vi "STED Control V11.vi"() -> ()   [LabVIEW 2014]
uses:
  Type Defs/Image Acquisition Parameters.ctl
  Laser Controls.ctl
  Detectors.ctl
  Type Defs/P541.ctl
  Type Defs/M227.ctl
  Type Defs/P612.ctl
  Type Defs/M686.ctl
  Type Defs/P841.ctl
  Type Defs/ASI.ctl
  Type Defs/N664_V2.ctl
  Type Defs/STED Graph Controls.ctl
  Type Defs/Display Controls.ctl
  FPGA-7842R-Reference.ctl
  Manual Controls V2.ctl
  Scan Parameters.ctl
  <vilib>/Utility/miscctls.llb/LVPositionTypeDef.ctl
  Focus Lock/Controls/Counter Action.ctl
  Controls/StageStates.ctl
  Focus Lock/Controls/Standard Action for Focus Lock.ctl
  <vilib>/Utility/miscctls.llb/LVRectTypeDef.ctl
  <vilib>/event_ctls.llb/lveventtype.ctl
  <vilib>/Utility/file.llb/Read From Spreadsheet File (DBL).vi
  <vilib>/Utility/file.llb/Write To Spreadsheet File (DBL).vi
panel:
  out "Graph Ref Out":refnum<vi>[](array[refnum])
  out "Frame Counter":i32
  in  "Follow Cursor":bool
  in  "Laser Controls 2":T1={"Laser On Time (Ticks)"=16, "Laser Delay (Ticks)"=3}
  out "Channel 6":sgl[][](graph)
  out "Channel 5":sgl[][](graph)
  out "Channel 4":sgl[][](graph)
  out "Channel 3":sgl[][](graph)
  out "Channel 2":sgl[][](graph)
  out "Channel 1":sgl[][](graph)
  in  "Display Controls":T2
  in  "Graph Tools":T3={"Zoom Out"=FALSE, "Zoom In"=FALSE, "Reset Zoom"=FALSE, "Pan Tool"=FALSE, "Show Cursor"=FALSE, "Load File"=FALSE, "Fit Tool"=FALSE, "Smooth Tool"=FALSE, "Merge Tool"=FALSE, "Auto Scale"=FALSE, "Apply Color"=FALSE, "Color Map"=enum."Fire"}
  in  "Shutters":T4
  in  "Upper Objective Z - N664":T5={"Up N664"=FALSE, "Down N664"=FALSE, "Step Size (um)"=0.001, "Position (mm)"=0.0, "Home"=FALSE, "Save"=FALSE} {"Step Size (um)" min=0.001}
  in  "Cavity Translation Z - ASI":T6={"Up ASI"=FALSE, "Down ASI"=FALSE, "Step Size (um)"=0.001, "Z (um)"=0.001, "F (um)"=0.001, "Velocity"=0.001} caption="ASI" {"Velocity" min=0.001; "F (um)" min=0.001; "Z (um)" min=-1500.0 max=1500.0; "Step Size (um)" min=0.001}
  in  "Phase Comp Mirror - P841":T7={"Position (µm)"=0.0, "Step Size (µm)"=0.05, "Up P841"=FALSE, "Down P841"=FALSE}
  in  "Sample Stage XY - M686":T8={"Home Button"=FALSE, "Up Button"=FALSE, "Left Button"=FALSE, "Down Button"=FALSE, "Right Button"=FALSE, "X"=0.0, "Y"=0.0, "Step Size (um)"=1.0} {"Y" format="%#_8g"; "X" format="%#_8g"}
  in  "Bottom Objective XY - P612":T9
  in  "Abort AllStage":bool
  in  "Stages":T10={"M227"=TRUE, "N664"=TRUE, "P612"=TRUE, "M686"=TRUE, "P841"=TRUE, "ASI"=FALSE}
  in  "Sample Z Coarse - M227":T11
  in  "Tab Control":T12(tab)
  in  "SLM":bool
  in  "DM":bool
  in  "Timing":bool
  in  "Focus Lock":bool
  in  "Stage Monitor":bool
  in  "Camera":bool
  in  "Sample Z - P541":T13={"Step Up"=FALSE, "Step Down"=FALSE, "Z Position"=0.0, "Step Size (um)"=1.0, "Home"=FALSE, "Save"=FALSE}
  in  "Detectors":T14={"PMT"=TRUE, "Far Red (685/40 nm)"=FALSE, "Orange (624/40 nm)"=FALSE, "Green (525/50 nm)"=FALSE, "Sum All"=FALSE}
  in  "Laser Controls":T15 {"STED Power (V)" scale=0.0..10.0}
  in  "Save File Path":path=path "C:/isoSTED_Data/Temp/Test_0000.dbl"
  in  "Capture":bool
  in  "Image Acquisition Parameters":T16={"Scan Type"=enum."Beam Scanning", "Scan Mode"=enum."XY", "Fast Axis Frequency (Hz)"=15780.0, "Image Format"=256, "Line Accumulations"=100, "Frames Per Capture"=1, "Frames Accumulations"=1, "Image Dimension (um)"=[15.0, 15.0], "Number of Z Steps"=1, "Z Steps Size (um)"=1.0, "Pixel Size (nm)"=[58.59375, 58.59375], "Customized Image Format"=[]} {"Z Steps Size (um)" min=0.0; "Number of Z Steps" min=1; "Frames Accumulations" min=1; "Frames Per Capture" min=1; "Line Accumulations" min=1; "Image Format" items=["64 x 64"=64, "128 x 128"=128, "256 x 256"=256, "512 x 512"=512, "1024 x 1024"=1024, "2048 x 2048"=2048, "Customized..."=0]}
  in  "Live":bool
  in  "Exit":bool
  # "Length"
  # "Height"
  # "XY"
  # "Z"
  # "Length"
  # "Height"
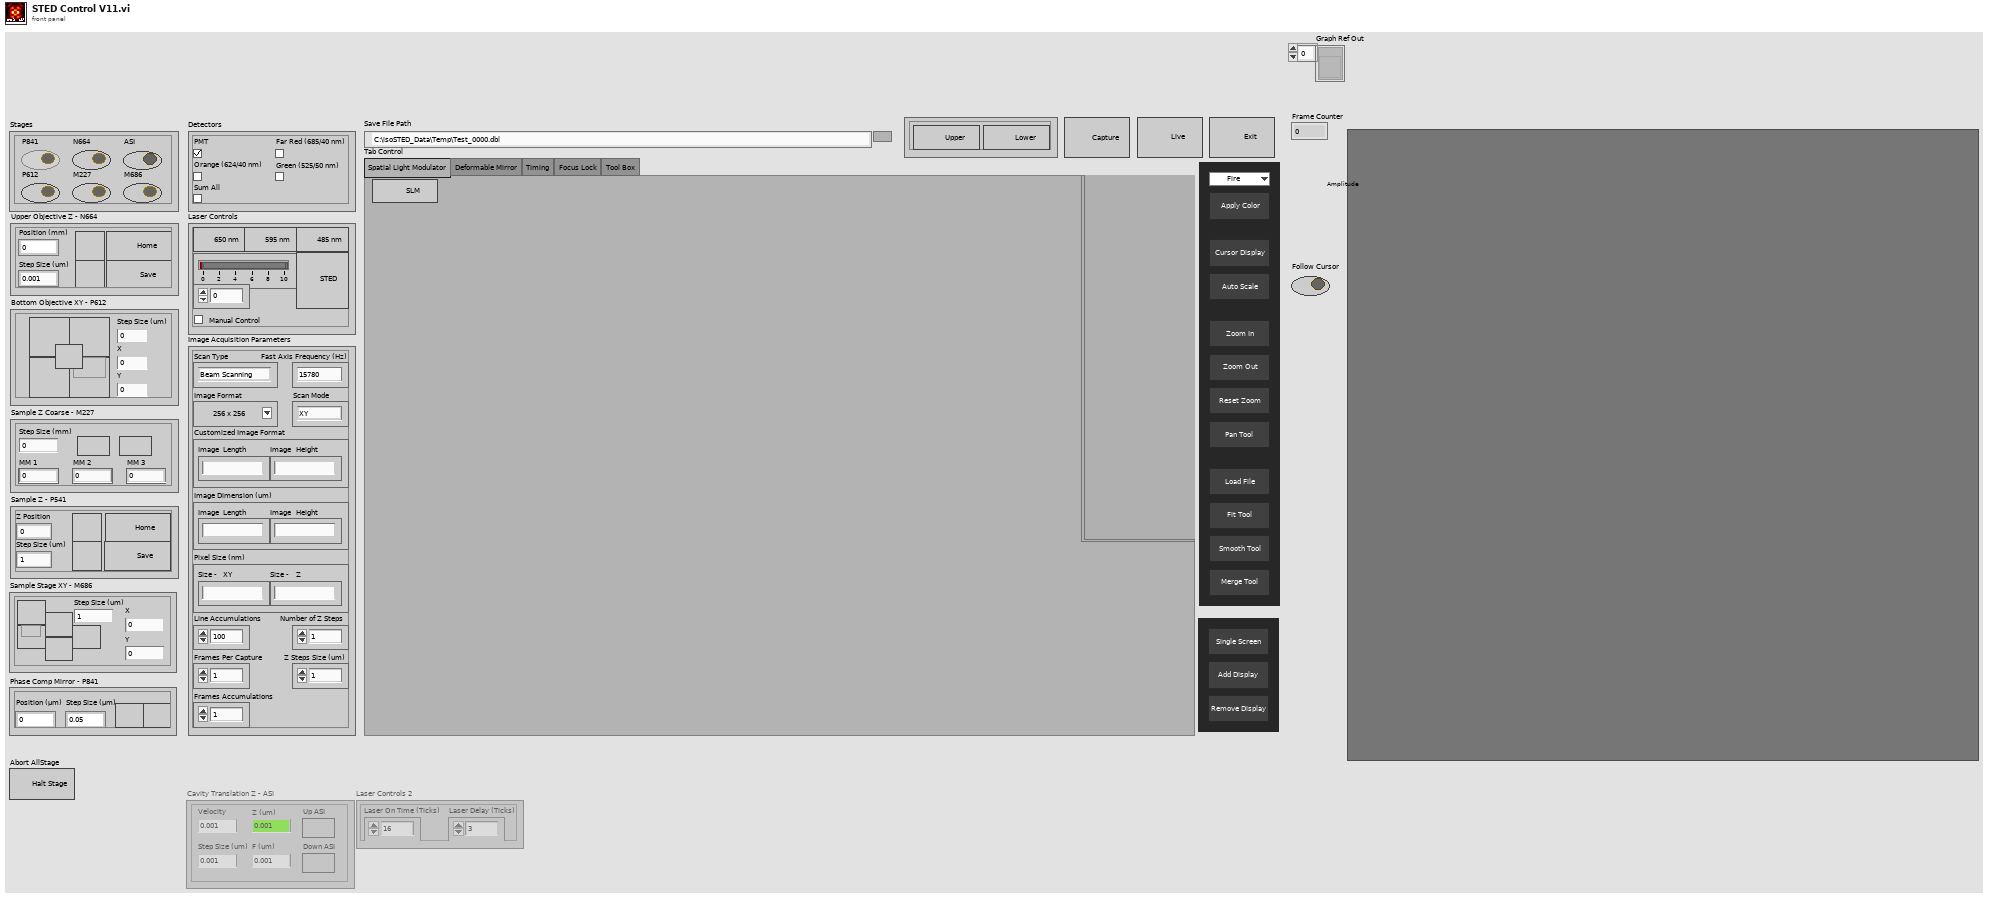
[diagram p1: front panel]
types:
  T1 = cluster{"Laser On Time (Ticks)":i8, "Laser Delay (Ticks)":i8}
  T2 = typedef "Display Controls.ctl" = cluster{"Remove Display":bool, "Add Display":bool, "Single Screen":bool}
  T3 = typedef "STED Graph Controls.ctl" = cluster{"Zoom Out":bool, "Zoom In":bool, "Reset Zoom":bool, "Pan Tool":bool, "Show Cursor":bool, "Load File":bool, "Fit Tool":bool, "Smooth Tool":bool, "Merge Tool":bool, "Auto Scale":bool, "Apply Color":bool, "Color Map":enum16{"System", "Fire", "Gray", "Red", "Green", "Blue", "Cyan", "Magenta", "Yellow", "Red-White", "Green-White", "Blue-White", "Glow"}}
  T4 = cluster{"Upper Shutter":bool, "Lower Shutter":bool}
  T5 = typedef "N664_V2.ctl" = cluster{"Up N664":bool, "Down N664":bool, "Step Size (um)":dbl, "Position (mm)":dbl, "Home":bool, "Save":bool}
  T6 = typedef "ASI.ctl" = cluster{"Up ASI":bool, "Down ASI":bool, "Step Size (um)":dbl, "Z (um)":dbl, "F (um)":dbl, "Velocity":dbl}
  T7 = typedef "P841.ctl" = cluster{"Position (µm)":dbl, "Step Size (µm)":dbl, "Up P841":bool, "Down P841":bool}
  T8 = typedef "M686.ctl" = cluster{"Home Button":bool, "Up Button":bool, "Left Button":bool, "Down Button":bool, "Right Button":bool, "X":dbl, "Y":dbl, "Step Size (um)":dbl}
  T9 = typedef "P612.ctl" = cluster{"Home Button":bool, "Up Button":bool, "Left Button":bool, "Down Button":bool, "Right Button":bool, "Step Size (um)":dbl, "X":dbl, "Y":dbl}
  T10 = cluster{"M227":bool, "N664":bool, "P612":bool, "M686":bool, "P841":bool, "ASI":bool}
  T11 = typedef "M227.ctl" = cluster{"Up M227":bool, "Down M227":bool, "Step Size (mm)":dbl, "MM 1":dbl, "MM 2":dbl, "MM 3":dbl}
  T12 = enum32{"Spatial Light Modulator", "Deformable Mirror", "Timing", "Focus Lock", "Tool Box"}
  T13 = typedef "P541.ctl" = cluster{"Step Up":bool, "Step Down":bool, "Z Position":dbl, "Step Size (um)":dbl, "Home":bool, "Save":bool}
  T14 = typedef "Detectors.ctl" = cluster{"PMT":bool, "Far Red (685/40 nm)":bool, "Orange (624/40 nm)":bool, "Green (525/50 nm)":bool, "Sum All":bool}
  T15 = typedef "Laser Controls.ctl" = cluster{"STED Power (V)":dbl, "STED":bool, "650 nm":bool, "590 nm":bool, "485 nm":bool, "Manual Control":bool}
  T16 = typedef "Image Acquisition Parameters.ctl" = cluster{"Scan Type":enum16{"Sample Scanning", "Beam Scanning"}, "Scan Mode":enum16{"XY", "XZ", "YZ", "XYZ"}, "Fast Axis Frequency (Hz)":dbl, "Image Format":u16, "Line Accumulations":u16, "Frames Per Capture":u16, "Frames Accumulations":u16, "Image Dimension (um)":dbl[], "Number of Z Steps":u8, "Z Steps Size (um)":dbl, "Pixel Size (nm)":dbl[], "Customized Image Format":dbl[]}
  T17 = typedef "Scan Parameters.ctl" = cluster{"Fast_Ax_Amp_V":dbl, "Fast_Ax_Off_V":dbl, "Slow_Ax_Amp_V":dbl, "Slow_Ax_Off_V ":dbl, "Slow_Ax_Max_V_VperS":dbl, "Slow_Ax1_Del25ns":i32, "Slow_Ax2_Del25ns":i32, "Stage_X_Off_V":dbl, "Stage_Y_Off_V":dbl, "Stage_Z_Off_V":dbl, "Galvo1_Off_V":dbl, "Galvo2_Off_V":dbl, "Last_Scan_Mode":enum16{"XY", "XZ", "YZ", "XYZ"}, "Current_Scan_Mode":enum16{"XY", "XZ", "YZ", "XYZ"}, "Fly_Back_Lines":u16, "Linear_Ramp_End":u32, "Z_Step_I16":i16, "Z_Start_I16":i16, "Laser_States _U32":u32, "590_Voltage_I16":i16, "775_AOM_Volt_I16":i16, "Blanking OFF":bool, "Unused_Axis_I16":i16}
  T18 = typedef "Manual Controls V2.ctl" = cluster{"Galvo 1 Position (I16)":i16, "Galvo 2 Position (I16)":i16, "X Axis Voltage (I16)":i16, "Y Axis Voltage (I16)":i16, "Z Axis Voltage (I16)":i16, "Res Mirror Amp (I16)":i16, "Res Mirror Mute":bool, "Upper Shutter":bool, "Lower Shutter":bool}
  T19 = typedef "FPGA-7842R-Reference.ctl" = enum16{"Stage Control", "Laser Control", "Unused Axis I16", "Exit", "Set Res Mirror", "Set Galvo", "Current Frame for Capture", "Default", "Close FPGA", "Stop Waveforms", "Start Waveforms", "Shutter Control", "Initialize"}
  T20 = typedef "Counter Action.ctl" = enum16{"Zero", "Plus One", "Read"}
  T21 = enum8{"Enabled", "Disabled", "Disabled and Grayed Out"}
  T22 = typedef "StageStates.ctl" = enum16{"POSITION", "MVR", "MOVE", "HALT", "ONTARGET", "ERROR", "EXIT", "HOME", "ZEROPOS", "NANOPOS", "QUIT", "ANALOG"}
  T23 = typedef "Standard Action for Focus Lock.ctl" = enum16{"Read", "Write"}
  T24 = typedef "LVRectTypeDef.ctl" = cluster{"Left":i16, "Top":i16, "Right":i16, "Bottom":i16}
  T25 = enum32{"Invalid", "Standard", "Closed", "Hidden", "Minimized", "Maximized"}
  T26 = typedef "lveventtype.ctl" = enum32{"Null", "Timeout", "Annotation Menu Selection", "Annotation Menu Selection?", "App Instance Close", "App Instance Close?", "Autoscale Range Change", "Bookmark Info Change", "Cell Edit", "Cell Edit?", "Cursor Grab", "Cursor Grab?", "Cursor Menu Selection", "Cursor Menu Selection?", "Cursor Move", "Cursor Release", "Data Change", "Direction Change", "Display State Change", "Drag Ended", "Drag Enter", "Drag Leave", "Drag Over", "Drag Source Update", "Drag Starting", "Drag Starting?", "Drop", "Exec State Change", "Key Down", "Key Down?", "Key Repeat", "Key Repeat?", "Key Up", "Listbox Double Click", "Menu Activation?", "Menu Selection (App)", "Menu Selection? (App)", "Menu Selection (User)", "Mouse Down", "Mouse Down?", "Mouse Enter", "Mouse Leave", "Mouse Move", "Mouse Up", "Mouse Wheel", "NI Security User Change (App)", "Pane Size", "Panel Close", "Panel Close?", "Panel Resize", "Plot Attribute Change", "Scale Range Change", "Shortcut Menu Activation?", "Shortcut Menu Selection (App)", "Shortcut Menu Selection? (App)", "Shortcut Menu Selection (User)", "Tree Double Click", "Tree Drag", "Tree Drag?", "Tree Drop", "Tree Drop?", "Tree Item Close", "Tree Item Close?", "Tree Item Open", "Tree Item Open?", "User Event", "Value Change"}
  T27 = typedef "LVPositionTypeDef.ctl" = cluster{"Left":i32, "Top":i32}
  T28 = cluster{"Upper Shutter":bool, "Upper Shutter":bool}
  T29 = cluster{bool, bool, dbl, "Numeric":dbl, "Numeric":dbl, "Numeric":dbl}
  T30 = cluster{"Down_N664":bool, "Down_N664":bool, "Step Size (um)":dbl, "Numeric":dbl, bool, bool}
  T31 = cluster{bool, bool, bool, bool, bool, dbl, "Numeric":dbl, "Numeric":dbl}
  T32 = cluster{bool, bool, bool, bool, bool, "Numeric":dbl, "Numeric":dbl, dbl}
  T33 = cluster{"Scan Type":bool, "Scan Mode":bool, "Fast Axis Frequency (Hz)":bool, "Image Format":bool, "Line Accumulations":bool, "Frames Per Capture":bool, "Frames Accumulations":bool, "Image Dimension (um)":bool[], "Number of Z Steps":bool, "Z Steps Size (um)":bool, "Pixel Size (nm)":bool[], "Customized Image Format":bool[]}
  T34 = typedef "Focus Lock.ctl" = cluster{"EXIT":bool, "Lock Current":bool, "Manual":bool, "Drift":bool, "Move":bool, "Control Option":bool}
  T35 = typedef "LVAllMonitorsDisplayTypeDef.ctl" = cluster{"Bounds":cluster{"Left":i16, "Top":i16, "Right":i16, "Bottom":i16}, "Depth":i16}[]
  T36 = cluster{"Bounds":cluster{"Left":i16, "Top":i16, "Right":i16, "Bottom":i16}, "Depth":i16}
  T37 = enum16{"System", "Fire", "Gray", "Red", "Green", "Blue", "Cyan", "Magenta", "Yellow", "Red-White", "Green-White", "Blue-White", "Glow"}
  T38 = typedef "LVPointDoubleTypeDef.ctl" = cluster{"Cursor X":dbl, "Cursor Y":dbl}
  T39 = typedef "LVRangeTypeDef.ctl" = cluster{"Minimum":dbl, "Maximum":dbl, "Increment":dbl, "Minor Increment":dbl, "Start":dbl}
  T40 = typedef "IMAQ Image.ctl" = refnum<image>
  T41 = typedef "Waveform Data.ctl" = cluster{"Waveform Scan Parameters":cluster{"Scanning Mode":u8, "Fast Axis WF Length (Elements)":i32, "Fast Axis Sample Period (Ticks)":u32, "Slow Axis 1 WF Length (Elements)":i32, "Slow Axis 1 Sample Period (Ticks)":u32, "Slow Axis 1 Delay (25 ns) Steps":i32, "Slow Axis 2 WFLength (Elements)":i32, "Slow Axis 2 Sample Period (Ticks)":u32, "Slow Axis 2 Delay (25 ns) Steps":i32}, "Fast Axis Waveform":dbl[], "Slow Axis 1 Waveform":dbl[], "Slow Axis 2 Waveform":dbl[]}
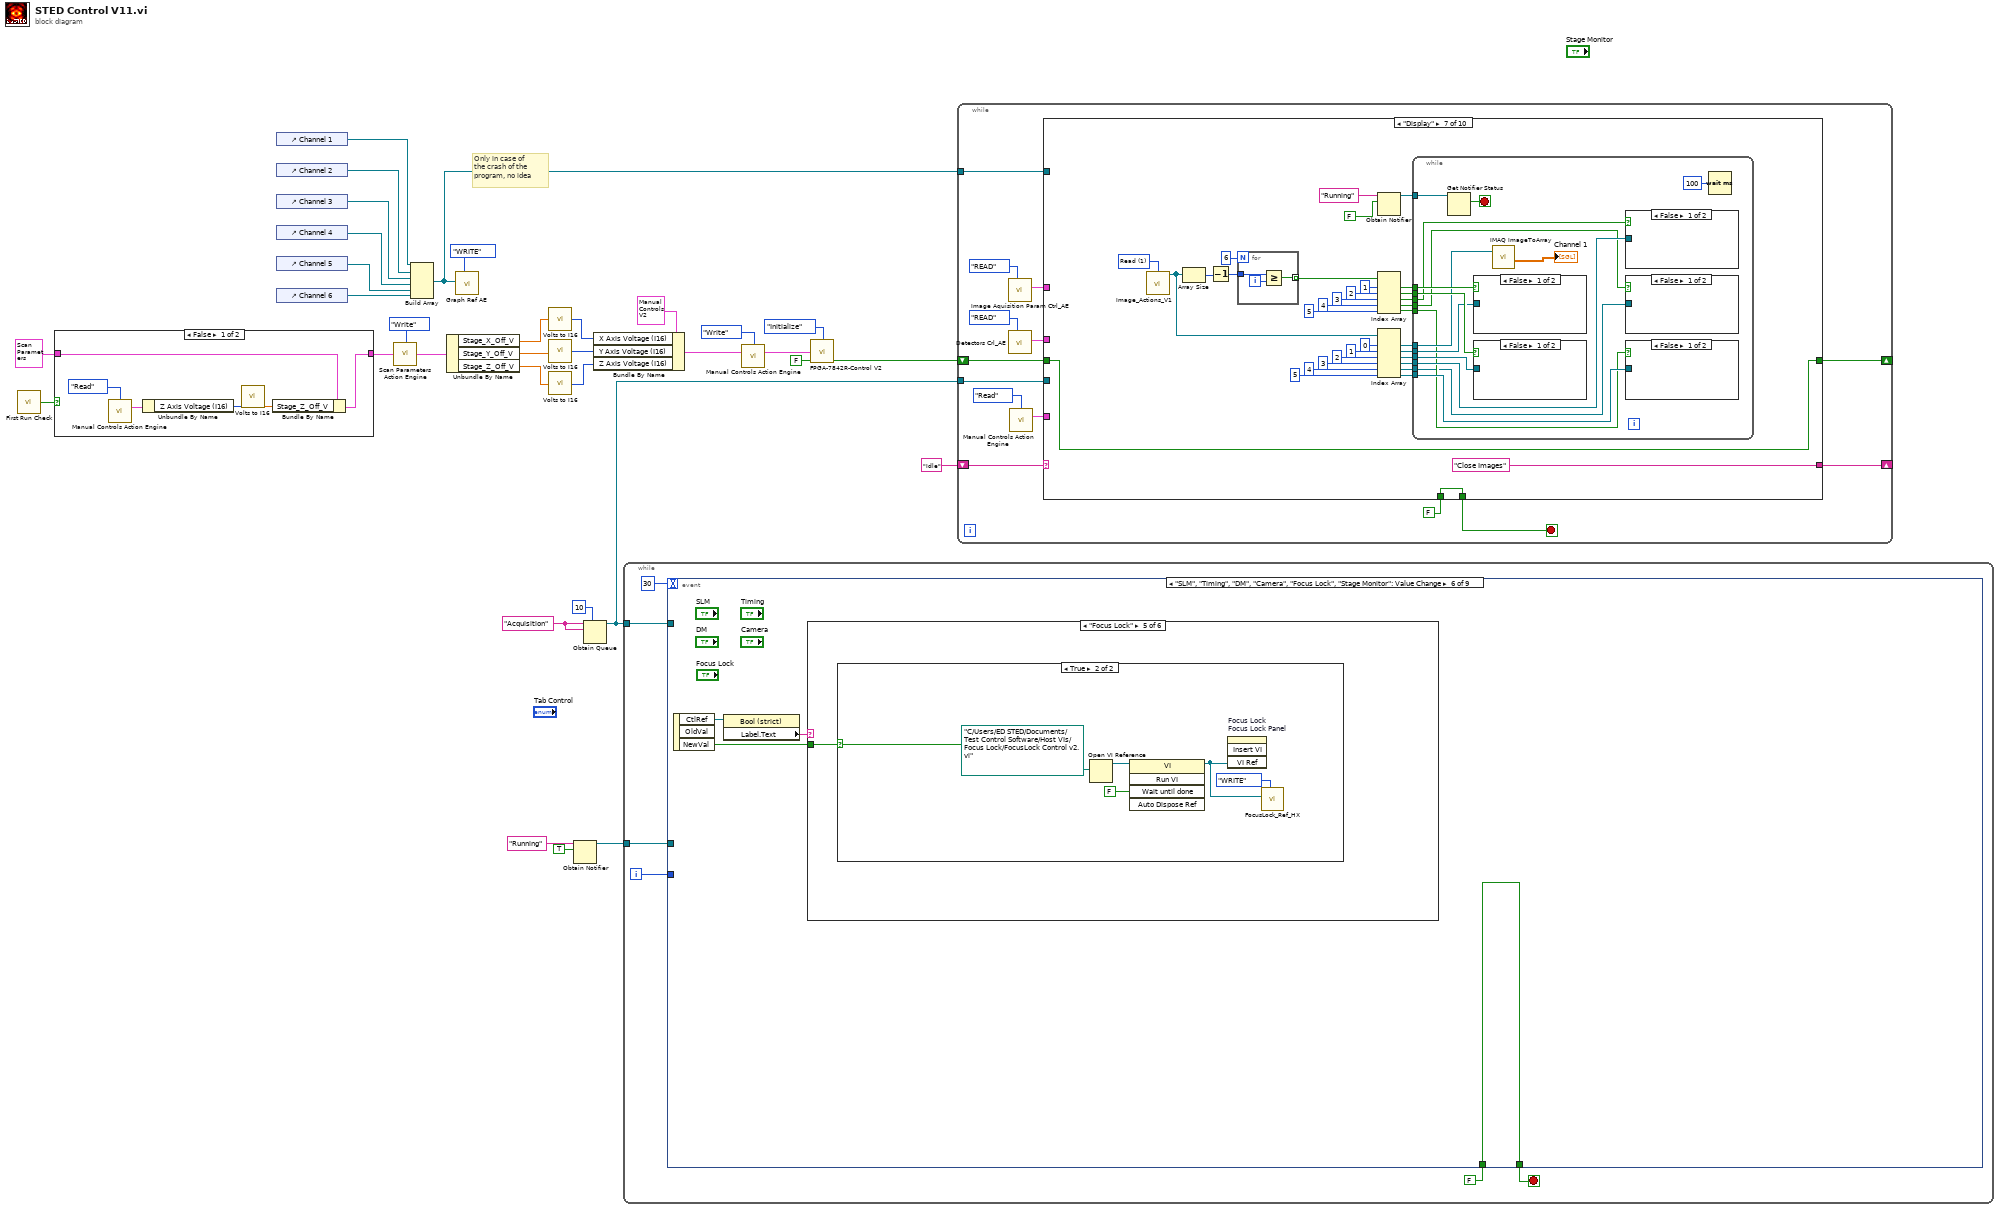
[diagram p0: block diagram]
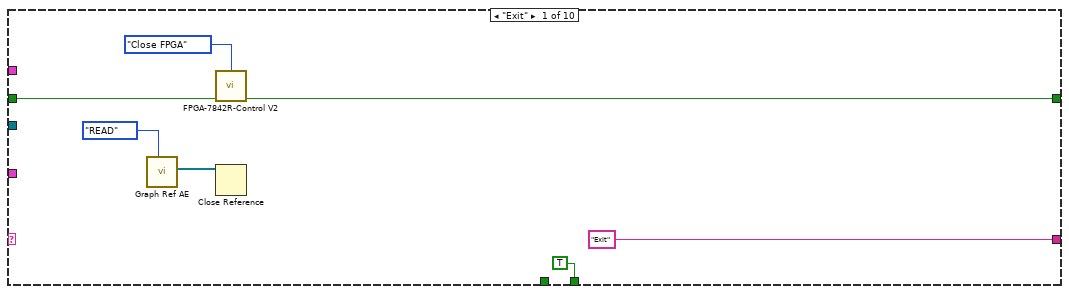
[diagram p3: hidden frame]
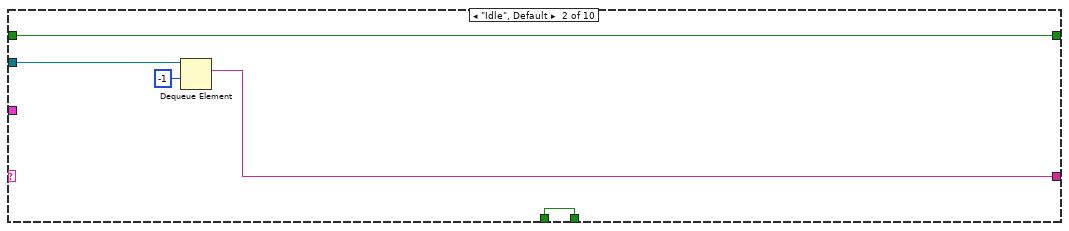
[diagram p4: hidden frame]
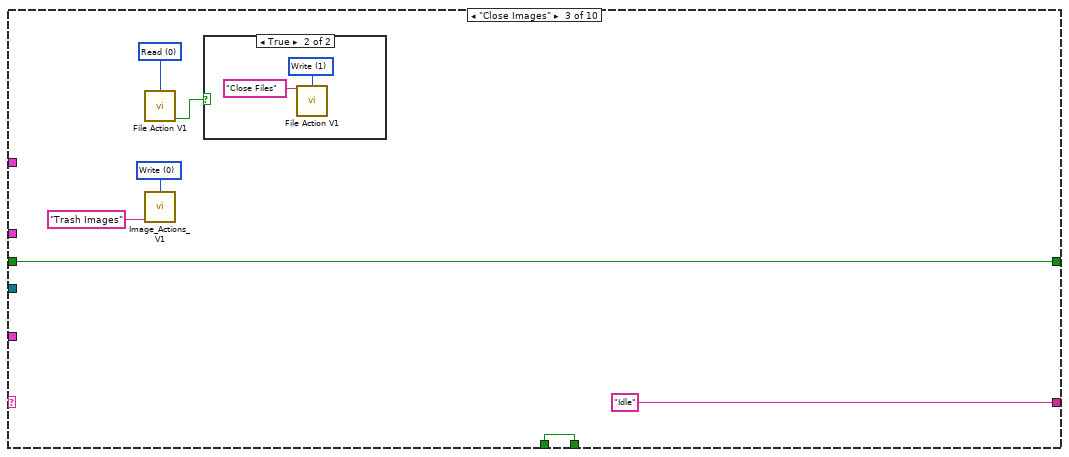
[diagram p5: hidden frame]
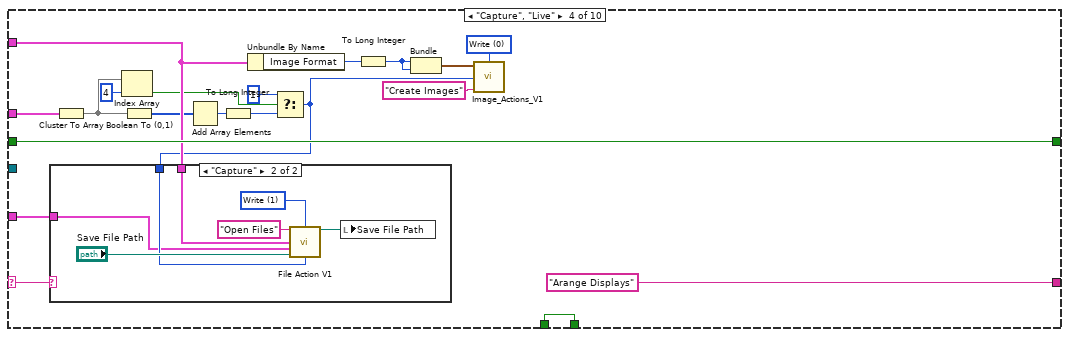
[diagram p7: hidden frame]
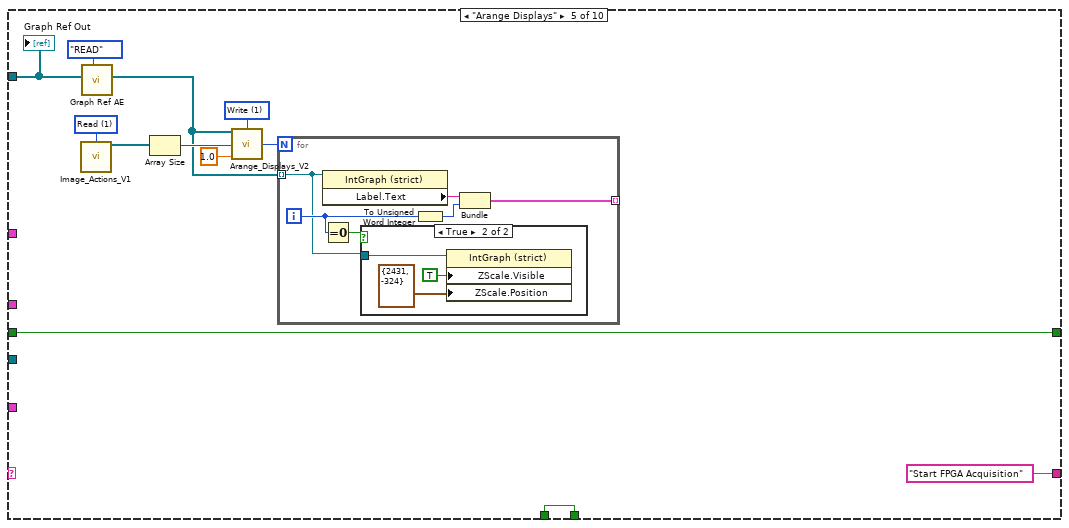
[diagram p9: hidden frame]
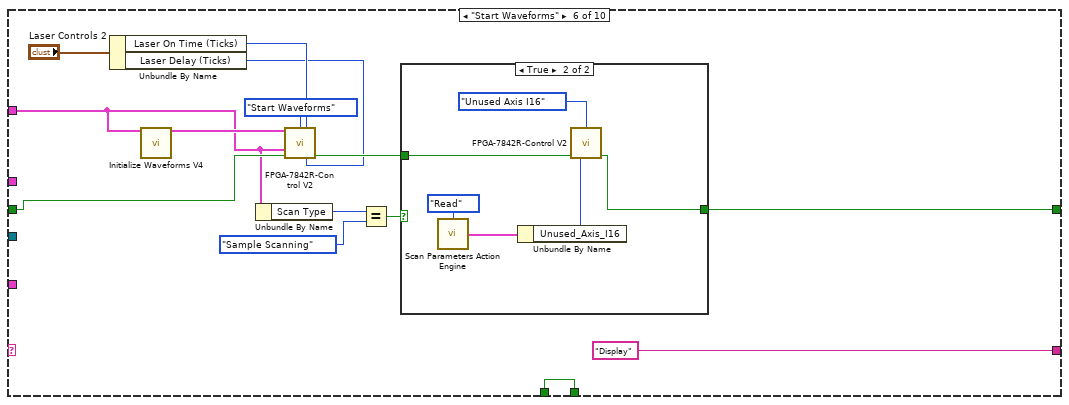
[diagram p11: hidden frame]
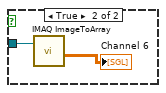
[diagram p13: hidden frame]
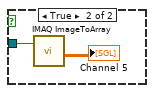
[diagram p14: hidden frame]
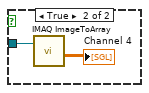
[diagram p15: hidden frame]
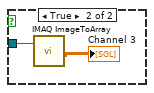
[diagram p16: hidden frame]
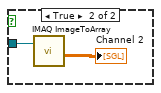
[diagram p17: hidden frame]
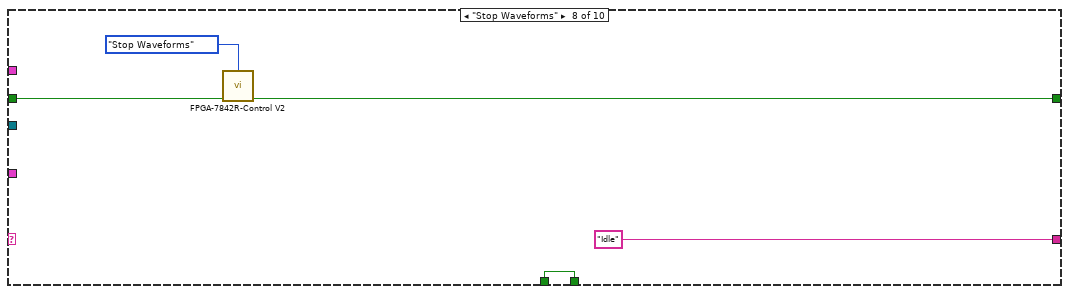
[diagram p18: hidden frame]
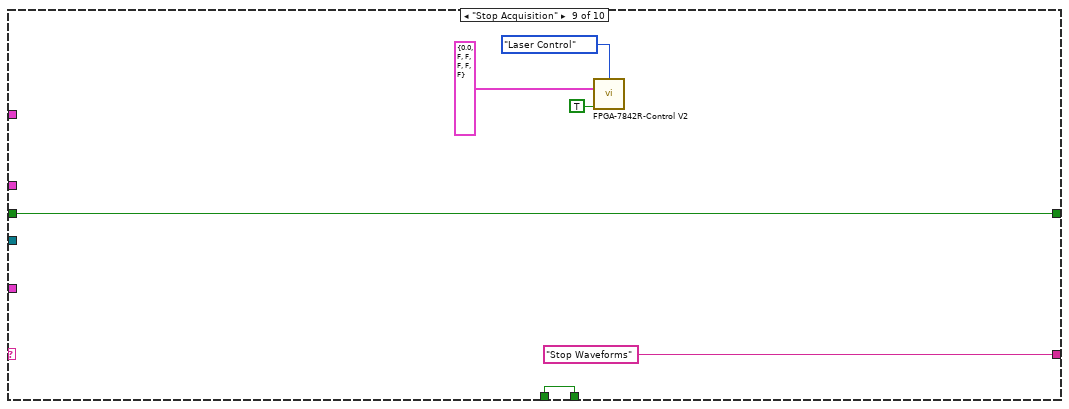
[diagram p19: hidden frame]
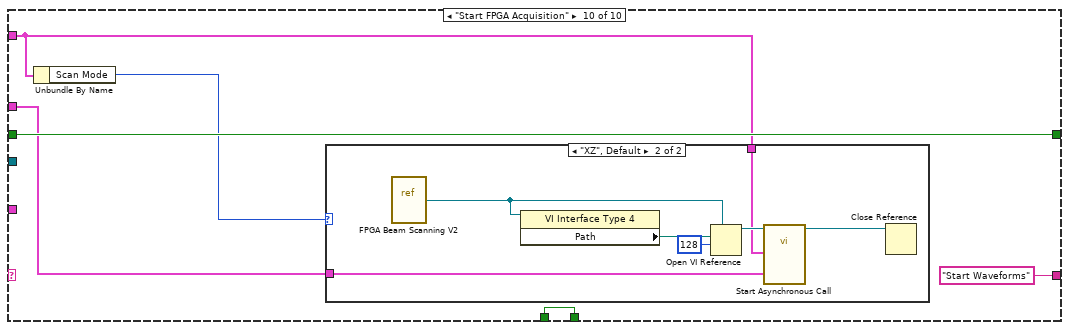
[diagram p20: hidden frame]
diagram:
  w16 = "Acquisition" ("name (unnamed)")
  # "Only in case of \nthe crash of the\nprogram, no idea"
  n1 = call "First Run Check.vi"() -> ("First Run?"=w10:bool)  [unwired: 15 in]
  n2 = case shown="False" w10 {
    tunnel: T17 {"Fast_Ax_Amp_V"=0.0, "Fast_Ax_Off_V"=0.0, "Slow_Ax_Amp_V"=0.0, "Slow_Ax_Off_V "=0.0, "Slow_Ax_Max_V_VperS"=0.0, "Slow_Ax1_Del25ns"=0, "Slow_Ax2_Del25ns"=0, "Stage_X_Off_V"=5.0, "Stage_Y_Off_V"=5.0, "Stage_Z_Off_V"=5.0, "Galvo1_Off_V"=0.0, "Galvo2_Off_V"=0.0, "Last_Scan_Mode"=enum."XY", "Current_Scan_Mode"=enum."XY", "Fly_Back_Lines"=0, "Linear_Ramp_End"=0, "Z_Step_I16"=0, "Z_Start_I16"=0, "Laser_States _U32"=0, "590_Voltage_I16"=0, "775_AOM_Volt_I16"=0, "Blanking OFF"=FALSE, "Unused_Axis_I16"=16384} ("Scan Parameters IN") -> [w39 w40]
    tunnel: [w34 w40] -> w8
    frame False {
      n3 = call "Manual Controls Action Engine.vi"("Action"=enum16{"Read", "Write"}."Read") -> ("Manual Controls Out"=w37:T18)  [unwired: 14 in]
      n4 = Unbundle By Name(w37) -> ("Z Axis Voltage (I16)"=w38:i16)
      n5 = call "Volts to I16.vi"("Volatge (I16)"=w38) -> ("Voltage (V)"=w35:dbl)  [unwired: 13 in, 1 out]
      n6 = Bundle By Name(cluster=w39, "Stage_Z_Off_V"=w35) -> (w34:T17)
    }
    frame True {
    }
  }
  n7 = control-ref of="Channel 1"() -> (w5:refnum<vi>)
  n8 = control-ref of="Channel 2"() -> (w6:refnum<vi>)
  n9 = control-ref of="Channel 3"() -> (w7:refnum<vi>)
  n10 = control-ref of="Channel 4"() -> (w2:refnum<vi>)
  n11 = control-ref of="Channel 5"() -> (w4:refnum<vi>)
  n12 = control-ref of="Channel 6"() -> (w3:refnum<vi>)
  n13 = call "Scan Parameters Action Engine.vi"("Action"=enum16{"Read", "Write"}."Write", "Scan Parameters IN"=w8) -> ("Scan Parameters OUT"=w26:T17)  [unwired: 13 in]
  n14 = Build Array(w5, w6, w7, w2, w4, w3) -> (w1:refnum<vi>[])
  n15 = Unbundle By Name(w26) -> ("Stage_X_Off_V"=w22:dbl, "Stage_Y_Off_V"=w21:dbl, "Stage_Z_Off_V"=w20:dbl)
  n16 = call "Graph Ref AE.vi"("Action"=enum16{"READ", "WRITE"}."WRITE", "Graph Ref In"=w1) -> ()  [unwired: 9 in, 1 out]
  n17 = call "Volts to I16.vi"("Voltage (V)"=w22) -> ("I16"=w23:i16)  [unwired: 13 in, 1 out]
  n18 = call "Volts to I16.vi"("Voltage (V)"=w21) -> ("I16"=w24:i16)  [unwired: 13 in, 1 out]
  n19 = call "Volts to I16.vi"("Voltage (V)"=w20) -> ("I16"=w25:i16)  [unwired: 13 in, 1 out]
  n20 = Obtain Notifier(name (unnamed)="Running", notification data type=TRUE) -> (notifier out=w12:refnum<notifier>)  [unwired: 2 in, 2 out]
  n21 = Obtain Queue(max queue size (-1, unlimited)=10, name (unnamed)=w16, element data type=w16) -> (queue out=w18:refnum<queue>)  [unwired: 2 in, 2 out]
  n22 = Bundle By Name(cluster=T18 {"Galvo 1 Position (I16)"=-280, "Galvo 2 Position (I16)"=0, "X Axis Voltage (I16)"=16384, "Y Axis Voltage (I16)"=16384, "Z Axis Voltage (I16)"=16384, "Res Mirror Amp (I16)"=0, "Res Mirror Mute"=FALSE, "Upper Shutter"=FALSE, "Lower Shutter"=FALSE} ("Manual Controls"), "X Axis Voltage (I16)"=w23, "Y Axis Voltage (I16)"=w24, "Z Axis Voltage (I16)"=w25) -> (w27:T18)
  n23 = while {
    tunnel: w18 -> [w44]
    tunnel: w12 -> [w41]
    i -> [w42]
    stop <- w46 stop-if-true
    n24 = event shown="[5] \"SLM\", \"Timing\", \"DM\", \"Camera\", \"Focus Lock\", \"Stage Monitor\": Value Change" {
      selector: _ -> [_ _ _ _ _ _ _ _ _]
      dyn-events: _ -> [_ _ _ _ _ _ _ _ _]
      timeout: 30 -> [_ _ _ _ _ _ _ _ _]
      tunnel: [w54 w198 w224 w389 _ w736 w831 w1035 w1088] -> w46
      tunnel: FALSE -> [w54 w198 w224 w389 _ w736 w831 w1035 _]
      tunnel: w44 -> [w51 w197 _ _ _ _ _ _ w1087]
      tunnel: w42 -> [w49 _ _ _ _ _ _ _ _]
      tunnel: w41 -> [w47 w195 _ _ _ _ _ _ w1081]
      event Timeout {
        n25 = event-data() -> ()  [unwired: 1 in, 3 out]
        n26 = Equal To 0?(x=w49) -> (x = 0?=w48:bool)
        n27 = Get Notifier Status(notifier=w47) -> (current notification=w53:bool)  [unwired: 1 in, 4 out]
        n28 = case shown="False" w48 {
          frame False {
            w55 = enum16{"WRITE", "READ", "HOME", "SAVE HOME"}."READ" ("Enum")
            n29 = call "Image Aquisition Param Ctrl_AE.vi"("Action"=enum16{"READ", "WRITE"}."READ") -> ("Image Acquisition Parameters Out"=w91:T16)  [unwired: 10 in]
            n30 = call "Detectors Crl_AE.vi"("Action"=enum16{"READ", "WRITE"}."READ") -> ("Detectors Parameters Out"=w92:T14)  [unwired: 10 in]
            n31 = call "LASERs_ Crl_AE.vi"("Action"=enum16{"READ", "WRITE"}."READ") -> ("Detectors Parameters Out"=w93:T15)  [unwired: 10 in]
            n32 = call "Frame Counter.vi"("Action"=Counter_Action."Read") -> ("Num"=→"Frame Counter":i32)
            n33 = local write "Image Acquisition Parameters"(w91) -> ()
            n34 = local write "Detectors"(w92) -> ()
            n35 = local write "Laser Controls"(w93) -> ()
            n36 = call "Stage_position_ae.vi"("StageID"="M686", "Enum"=w55) -> ("Position Out"=w66:dbl[])  [unwired: 8 in, 1 out]
            n37 = call "Stage_position_ae.vi"("StageID"="M227", "Enum"=w55) -> ("Position Out"=w73:dbl[])  [unwired: 8 in, 1 out]
            n38 = call "Stage_position_ae.vi"("StageID"="N664", "Enum"=w55) -> ("Position Out"=w58:dbl[])  [unwired: 8 in, 1 out]
            n39 = call "Stage_position_ae.vi"("StageID"="P841", "Enum"=w55) -> ("Position Out"=w81:dbl[])  [unwired: 8 in, 1 out]
            n40 = call "Stage_position_ae.vi"("StageID"="P612", "Enum"=w55) -> ("Position Out"=w56:dbl[])  [unwired: 8 in, 1 out]
            n41 = Index Array(array=w58, index=0) -> (element=w76:dbl)
            n42 = Index Array(array=w81, index=0) -> (element=w78:dbl)
            n43 = Index Array(array=w56, index #1=0 ("index"), index #2=1 ("index"), index #3=2 ("index")) -> (element #1=w87:dbl, element #2=w84:dbl, element #3=w82:dbl)
            n44 = Index Array(array=w66, index #1=0 ("index"), index #2=1 ("index")) -> (element #1=w63:dbl, element #2=w62:dbl)
            n45 = Index Array(array=w73, index #1=0 ("index"), index #2=1 ("index"), index #3=2 ("index")) -> (element #1=w70:dbl, element #2=w69:dbl, element #3=w68:dbl)
            n46 = property on="Position (µm)" class="DigNum (strict)"("Value"=w78) -> ()  [unwired: 2 in, 2 out]
            n47 = property on="Position (mm)" class="DigNum (strict)"("Value"=w76) -> ()  [unwired: 2 in, 2 out]
            n48 = property on="X" class="DigNum (strict)"("Value"=w87) -> ()  [unwired: 2 in, 2 out]
            n49 = property on="Y" class="DigNum (strict)"("Value"=w84) -> ()  [unwired: 2 in, 2 out]
            n50 = property on="X" class="DigNum (strict)"("Value"=w63) -> ()  [unwired: 2 in, 2 out]
            n51 = property on="MM 1" class="DigNum (strict)"("Value"=w70) -> ()  [unwired: 2 in, 2 out]
            n52 = property on="MM 2" class="DigNum (strict)"("Value"=w69) -> ()  [unwired: 2 in, 2 out]
            n53 = property on="Z Position" class="DigNum (strict)"("Value"=w82) -> ()  [unwired: 2 in, 2 out]
            n54 = property on="Y" class="DigNum (strict)"("Value"=w62) -> ()  [unwired: 2 in, 2 out]
            n55 = property on="MM 3" class="DigNum (strict)"("Value"=w68) -> ()  [unwired: 2 in, 2 out]
          }
          frame True {
            w95 = FALSE ("SLM")
            w97 = enum16{"WRITE", "READ", "HOME", "SAVE HOME"}."SAVE HOME" ("Enum")
            w109 = FALSE ("Upper Shutter")
            n56 = local read "Image Acquisition Parameters"() -> (w116:T16)
            n57 = local read "Laser Controls"() -> (w114:T15)
            n58 = local read "Detectors"() -> (w113:T14)
            n59 = Bundle("Upper Shutter"=w109, "Upper Shutter"=w109) -> (w110:T28)  [unwired: 1 in]
            n60 = property on="Shutters" class="Clust (strict)"("Value"=w110) -> ()  [unwired: 2 in, 2 out]
            n61 = call "Image Aquisition Param Ctrl_AE.vi"("Action"=enum16{"READ", "WRITE"}."WRITE", "Image Acquisition Parameters In"=w116) -> ()  [unwired: 9 in, 1 out]
            n62 = call "Detectors Crl_AE.vi"("Action"=enum16{"READ", "WRITE"}."WRITE", "Detectors Parameters In"=w113) -> ()  [unwired: 9 in, 1 out]
            n63 = call "LASERs_ Crl_AE.vi"("Action"=enum16{"READ", "WRITE"}."WRITE", "Detectors Parameters In"=w114) -> ()  [unwired: 9 in, 1 out]
            n64 = property on="Stages" class="Clust (strict)"() -> ("Controls[]"=w111:refnum<vi>[])  [unwired: 2 in, 2 out]
            n65 = for {
              tunnel: w111 -> [w121] mode=indexing
              n66 = property class="Ctl"(reference=w121) -> ("Label.Text"=w119:string, "Value"=w123:variant)  [unwired: 1 in, 2 out]
              n67 = Variant To Data(type=TRUE, Variant=w123) -> (data=w120:bool)  [unwired: 1 in, 1 out]
              n68 = call "All_Stages_Aloha.vi"("Aloha"=w120, "Stage ID"=w119) -> ("Position Out"=w118:dbl[])  [unwired: 9 in]
              n69 = case shown="\"M686\"" w119 {
                tunnel: w118 -> [_ w130 w138 w145 w154 w165 w175]
                frame "0", Default {
                }
                frame "M227" {
                  w134 = FALSE
                  n70 = Index Array(array=w130, index #1=0 ("index"), index #2=1 ("index"), index #3=2 ("index")) -> (element #1=w126:dbl, element #2=w125:dbl, element #3=w124:dbl)
                  n71 = Bundle(w134, w134, 0.0, "Numeric"=w126, "Numeric"=w125, "Numeric"=w124) -> (w132:T29)  [unwired: 1 in]
                  n72 = To Variant(anything=w132) -> (Variant=w131:variant)
                  n73 = property on="Sample Z Coarse - M227" class="Clust"("Value"=w131) -> ()  [unwired: 2 in, 2 out]
                }
                frame "N664" {
                  w135 = FALSE
                  w141 = FALSE ("Down_N664")
                  n74 = Index Array(array=w138, index=0) -> (element=w139:dbl)
                  n75 = Bundle("Down_N664"=w141, "Down_N664"=w141, "Step Size (um)"=1.0, "Numeric"=w139, w135, w135) -> (w137:T30)  [unwired: 1 in]
                  n76 = To Variant(anything=w137) -> (Variant=w136:variant)
                  n77 = property on="Upper Objective Z - N664" class="Clust"("Value"=w136) -> ()  [unwired: 2 in, 2 out]
                }
                frame "P612" {
                  w153 = FALSE
                  n78 = Index Array(array=w145, index #1=0, index #2=1, index #3=2 ("index")) -> (element #1=w150:dbl, element #2=w148:dbl, element #3=w143:dbl)
                  n79 = Bundle(w153, w153, w153, w153, w153, 1.0, "Numeric"=w150, "Numeric"=w148) -> (w149:T31)  [unwired: 1 in]
                  n80 = To Variant(anything=w149) -> (Variant=w144:variant)
                  n81 = property on="Bottom Objective XY - P612" class="Clust"("Value"=w144) -> ()  [unwired: 2 in, 2 out]
                  n82 = property on="Z Position" class="DigNum (strict)"("Value"=w143) -> ()  [unwired: 2 in, 2 out]
                }
                frame "M686" {
                  w163 = FALSE
                  n83 = Index Array(array=w154, index #1=0, index #2=1) -> (element #1=w158:dbl, element #2=w157:dbl)
                  n84 = Bundle(w163, w163, w163, w163, w163, "Numeric"=w158, "Numeric"=w157, 1.0) -> (w161:T32)  [unwired: 1 in]
                  n85 = To Variant(anything=w161) -> (Variant=w159:variant)
                  n86 = property on="Sample Stage XY - M686" class="Clust"("Value"=w159) -> ()  [unwired: 2 in, 2 out]
                  n87 = call "M686_timer.vi"("Reset"=TRUE) -> ()  [unwired: 1 out]
                }
                frame "P841" {
                  n88 = Index Array(array=w165, index=0) -> (element=w164:dbl)
                  n89 = property on="Position (µm)" class="DigNum (strict)"("Value"=w164) -> ()  [unwired: 2 in, 2 out]
                }
                frame "ASI" {
                  w171 = FALSE
                  n90 = Add Array Elements(numeric array=w175) -> (sum=w177:dbl)
                  n91 = Index Array(array=w175, index #1=0 ("index"), index #2=1 ("index")) -> (element #1=w170:dbl, element #2=w169:dbl)
                  n92 = Divide(x=w177, y=2000.0) -> ()  [unwired: 1 out]
                  n93 = Bundle By Name(cluster=T6 {"Up ASI"=FALSE, "Down ASI"=FALSE, "Step Size (um)"=0.001, "Z (um)"=0.001, "F (um)"=0.001, "Velocity"=0.001} ("Cavity Translation Z - ASI"), "Up ASI"=w171, "Down ASI"=w171, "Step Size (um)"=1.0, "Z (um)"=w170, "F (um)"=w169, "Velocity"=0.1) -> (w167:T6)
                  n94 = To Variant(anything=w167) -> (Variant=w168:variant)
                  n95 = property on="Cavity Translation Z - ASI" class="Clust"("Value"=w168) -> ()  [unwired: 2 in, 2 out]
                }
              }
            }
            n96 = call-poly <vilib>:"Read From Spreadsheet File.vi"("format (%.3f)"="%.4f", "number of rows (all:-1)"=1, "file path (dialog if empty)"=path "C:/Users/ED STED/Documents/Test Control Software/Host VIs/Stages/Stage Positions/home position.csv") -> ("first row"=w106:dbl[])  [unwired: 4 in, 4 out]
            n97 = Index Array(array=w106, index #1=0 ("index"), index #2=1 ("index")) -> (element #1=w102:dbl, element #2=w103:dbl)
            n98 = Build Array(w102) -> (w101:dbl[])
            n99 = Build Array(w103) -> (w99:dbl[])
            n100 = call "Stage_position_ae.vi"("Position In"=w101, "StageID"="P541", "Enum"=w97) -> ()  [unwired: 7 in, 2 out]
            n101 = call "Stage_position_ae.vi"("Position In"=w99, "StageID"="N664", "Enum"=w97) -> ()  [unwired: 7 in, 2 out]
            n102 = local write "Focus Lock"(w95) -> ()
            n103 = local write "SLM"(w95) -> ()
            n104 = local write "Timing"(w95) -> ()
            n105 = local write "DM"(w95) -> ()
            n106 = local write "Camera"(w95) -> ()
            n107 = call "Frame Counter.vi"("Action"=Counter_Action."Zero") -> ()  [unwired: 1 out]
          }
        }
        n108 = local read "Capture"() -> (w52:bool)
        n109 = And(x=w53, y=w52) -> (x .and. y?=w50:bool)
        n110 = case shown="False" w50 {
          tunnel: w51 -> [_ w183]
          frame False {
          }
          frame True {
            w181 = T21."Enabled" ("Disabled")
            n111 = local write "Capture"(FALSE ("Capture")) -> ()
            n112 = call "Frame Counter.vi"("Action"=Counter_Action."Zero") -> ()  [unwired: 1 out]
            n113 = Enqueue Element(queue=w183, element="Stop Acquisition" ("f")) -> ()  [unwired: 2 in, 3 out]
            n114 = property on="Live" class="Bool (strict)"("DisabledEnum"=w181) -> ()  [unwired: 2 in, 2 out]
            n115 = property on="Exit" class="Bool"("DisabledEnum"=w181) -> ()  [unwired: 2 in, 2 out]
          }
        }
      }
      event "Live", "Capture": Value Change {
        w187 = FALSE ("element")
        n116 = event-data() -> ("CtlRef"=w196:refnum<vi>, "NewVal"=w194:bool)  [unwired: 1 in]
        n117 = call "Detectors Crl_AE.vi"() -> ("Detectors Parameters Out"=w193:T14)  [unwired: 11 in]
        n118 = Unbundle By Name(w193) -> ("PMT"=w192:bool, "Far Red (685/40 nm)"=w191:bool, "Orange (624/40 nm)"=w190:bool, "Green (525/50 nm)"=w189:bool, "Sum All"=w188:bool)
        n119 = Build Array(w192, w191, w190, w189, w188, w187, w187, w187) -> (w186:bool[])
        n120 = Boolean Array To Number(Boolean array=w186) -> (number=w185:u32)
        n121 = case shown="1, Default" w185 {
          tunnel: w197 -> [_ w207]
          tunnel: w196 -> [_ w206]
          tunnel: w195 -> [_ w201]
          tunnel: w194 -> [_ w200]
          frame 0 {
            w199 = FALSE ("Live")
            n122 = call "Display Message to User"() -> ()  [unwired: 10 in, 2 out]
            n123 = local write "Capture"(w199) -> ()
            n124 = local write "Live"(w199) -> ()
          }
          frame 1, Default {
            n125 = Not(x=w200) -> (.not. x?=w204:bool)
            n126 = property class="Bool (strict)"(reference=w206) -> ("Label.Text"=w202:string)  [unwired: 1 in, 2 out]
            n127 = Send Notification(notification=w204, notifier=w201) -> ()  [unwired: 1 in, 2 out]
            n128 = Select(t=w202, s=w200, f="Stop Acquisition") -> (s? t:f=w203:string)
            n129 = case shown="\"Capture\"" w202 {
              tunnel: w200 -> [_ w209 w214]
              frame "False", Default {
              }
              frame "Live" {
                n130 = case shown="True" w209 {
                  tunnel: [T21."Enabled" ("Disabled") T21."Disabled and Grayed Out" ("Disabled")] -> w208
                  frame False {
                    n131 = call "Frame Counter.vi"("Action"=Counter_Action."Zero") -> ()  [unwired: 1 out]
                  }
                  frame True {
                    n132 = call "Frame Counter.vi"("Action"=Counter_Action."Zero") -> ()  [unwired: 1 out]
                  }
                }
                n133 = property on="Capture" class="Bool (strict)"("DisabledEnum"=w208) -> ()  [unwired: 2 in, 2 out]
                n134 = property on="Exit" class="Bool"("DisabledEnum"=w208) -> ()  [unwired: 2 in, 2 out]
              }
              frame "Capture" {
                n135 = case shown="False" w214 {
                  tunnel: [T21."Enabled" ("Disabled") T21."Disabled and Grayed Out" ("Disabled")] -> w215
                  frame False {
                    n136 = call "Frame Counter.vi"("Action"=Counter_Action."Zero") -> ()  [unwired: 1 out]
                  }
                  frame True {
                    n137 = call "Frame Counter.vi"("Action"=Counter_Action."Zero") -> ()  [unwired: 1 out]
                  }
                }
                n138 = property on="Live" class="Bool (strict)"("DisabledEnum"=w215) -> ()  [unwired: 2 in, 2 out]
                n139 = property on="Exit" class="Bool"("DisabledEnum"=w215) -> ()  [unwired: 2 in, 2 out]
              }
            }
            n140 = Enqueue Element(queue=w207, element=w203) -> ()  [unwired: 2 in, 3 out]
          }
        }
      }
      event "Shutters": Value Change {
        n141 = event-data() -> ("CtlRef"=w223:refnum<vi>, "NewVal"=w222:variant, "OldVal"=w221:variant)  [unwired: 1 in]
        n142 = property class="Clust"(reference=w223) -> ("Label.Text"=w220:string)  [unwired: 1 in, 2 out]
        n143 = case shown="\"Image Acquisition Parameters\"" w220 {
          tunnel: w222 -> [_ w239 _ _ _]
          tunnel: w221 -> [_ w237 _ _ _]
          frame Default {
          }
          frame "Image Acquisition Parameters" {
            n144 = Variant To Data(type="Image Acquisition Parameters", Variant=w239) -> (data=w236:T16)  [unwired: 1 in, 1 out]
            n145 = Variant To Data(type=w236, Variant=w237) -> (data=w235:T16)  [unwired: 1 in, 1 out]
            n146 = Not Equal?(x=w236, y=w235) -> (x != y?=w260:T33)
            n147 = Unbundle By Name(w260) -> ("Image Dimension (um)"=w245:bool[], "Image Format"=w243:bool, "Pixel Size (nm)"=w244:bool[], "Scan Mode"=w226:bool)
            n148 = Or Array Elements(Boolean array=w245) -> (logical OR=w249:bool)
            n149 = Or Array Elements(Boolean array=w244) -> (logical OR=w248:bool)
            n150 = Build Array(w249, w243, w248) -> (w247:bool[])
            n151 = Boolean Array To Number(Boolean array=w247) -> (number=w246:u32)
            n152 = case shown="1, 2" w246 {
              tunnel: w245 -> [_ w310 _]
              tunnel: w236 -> [w298 w303 w318]
              tunnel: [w298 w301 w316] -> w242
              tunnel: w244 -> [_ _ w315]
              tunnel: [w297 w300 w314] -> w241
              tunnel: [w296 w299 w313] -> w228
              frame 0, Default {
                n153 = Unbundle By Name(w298) -> ("Image Dimension (um)"=w297:dbl[], "Scan Mode"=w296:enum16{"XY", "XZ", "YZ", "XYZ"})
              }
              frame 1, 2 {
                # "Image Dimension or Format Change"
                n154 = Unbundle By Name(w303) -> ("Image Dimension (um)"=w309:dbl[], "Image Format"=w307:u16, "Scan Mode"=w299:enum16{"XY", "XZ", "YZ", "XYZ"})
                n155 = for {
                  tunnel: w310 -> [w312] mode=indexing
                  tunnel: w309 -> [w311] mode=indexing
                  tunnel: [w311] -> w308
                  stop <- w312 stop-if-true
                }
                n156 = To Double Precision Float(number=w307) -> (double precision float=w306:dbl)
                n157 = Build Array(w308, w308) -> (w300:dbl[])
                n158 = Divide(x=w300, y=w306) -> (x/y=w305:dbl[])
                n159 = Multiply(x=w305, y=1000.0) -> (x*y=w302:dbl[])
                n160 = Bundle By Name(cluster=w303, "Image Dimension (um)"=w300, "Pixel Size (nm)"=w302) -> (w301:T16)
              }
              frame 4 {
                # "Pixel Size Change"
                n161 = Unbundle By Name(w318) -> ("Pixel Size (nm)"=w324:dbl[], "Image Format"=w322:u16, "Scan Mode"=w313:enum16{"XY", "XZ", "YZ", "XYZ"})
                n162 = for {
                  tunnel: w315 -> [w326] mode=indexing
                  tunnel: w324 -> [w325] mode=indexing
                  tunnel: [w325] -> w323
                  stop <- w326 stop-if-true
                }
                n163 = Build Array(w323, w323) -> (w317:dbl[])
                n164 = To Double Precision Float(number=w322) -> (double precision float=w321:dbl)
                n165 = Multiply(x=w317, y=w321) -> (x*y=w320:dbl[])
                n166 = Multiply(x=w320, y=0.001) -> (x*y=w314:dbl[])
                n167 = Bundle By Name(cluster=w318, "Pixel Size (nm)"=w317, "Image Dimension (um)"=w314) -> (w316:T16)
              }
            }
            n168 = And(x=w226, y="Follow Cursor") -> (x .and. y?=w225:bool)
            n169 = case shown="True" w225 {
              tunnel: w228 -> [_ w270]
              frame False {
              }
              frame True {
                n170 = Not Equal?(x=w270, y=enum16{"XY", "XZ", "YZ", "XYZ"}."XZ") -> (x != y?=w268:bool)
                n171 = case shown="True" w268 {
                  frame False {
                    n172 = call "Y Slice.vi"() -> ("Y position"=w278:dbl)  [unwired: 1 in]
                    n173 = Build Array(0.0 ("element"), w278) -> (w276:dbl[])
                    n174 = call "AllStage_Limits_Array.vi"("Step(um)/Position(units)"=w276, "Axis"=bool[] [TRUE, TRUE, TRUE], "Stage ID"="M686", "MOVE/MVR"=enum16{"MOVE", "MVR"}."MVR") -> ("Positions"=w272:dbl[], "Boolean Array"=w273:bool[], "Stage ID"=w274:string)  [unwired: 4 in, 1 out]
                    n175 = call "AE_AllStages_Action V2.vi"("Velocity"=0.0, "Positions"=w272, "Axis"=w273, "Stage ID"=w274, "Action"=StageStates."MVR") -> ()  [unwired: 4 in, 3 out]
                  }
                  frame True {
                    n176 = call "Z Slice.vi"() -> ("Y position"=w292:dbl)  [unwired: 1 in]
                    n177 = call "Manual Controls Action Engine.vi"("Action"=enum16{"Read", "Write"}."Read") -> ("Manual Controls Out"=w287:T18)  [unwired: 14 in]
                    n178 = Multiply(x=w292, y=327.68) -> (x*y=w294:dbl)
                    n179 = Round To Nearest(number=w294) -> (nearest integer value=w293:dbl)
                    n180 = Unbundle By Name(w287) -> ("Z Axis Voltage (I16)"=w290:i16)
                    n181 = To Word Integer(number=w293) -> (16bit integer=w289:i16)
                    n182 = Add(x=w290, y=w289) -> (x+y=w288:i16)
                    n183 = Bundle By Name(cluster=w287, "Z Axis Voltage (I16)"=w288) -> (w286:T18)
                    n184 = call "Manual Controls Action Engine.vi"("Action"=enum16{"Read", "Write"}."Write", "Manual Controls In"=w286) -> ("Manual Controls Out"=w284:T18)  [unwired: 13 in]
                    n185 = call "FPGA-7842R-Control V2.vi"("Action"=FPGA-7842R-Reference."Stage Control", "Manual Controls"=w284, "Initialize"=TRUE) -> ()  [unwired: 11 in, 2 out]
                  }
                }
              }
            }
            n186 = Index Array(array=w241, index=0) -> (element=w265:dbl)
            n187 = Not Equal?(x=enum16{"XY", "XZ", "YZ", "XYZ"}."YZ" ("y"), y=w228) -> (x != y?=w250:bool)
            n188 = call "Res Mirror um to Volts.vi"("Image Size (um)"=w265) -> ("Voltage (V)"=w229:dbl)
            n189 = Select(t=15780.0, s=w250, f=200.0) -> (s? t:f=w253:dbl)
            n190 = In Range and Coerce(upper limit=5.0, x=w229, lower limit=0.0) -> (coerced(x)=w231:dbl)  [unwired: 1 out]
            n191 = call "Scan Parameters Action Engine.vi"("Action"=enum16{"Read", "Write"}."Read") -> ("Scan Parameters OUT"=w232:T17)  [unwired: 14 in]
            n192 = Bundle By Name(cluster=w232, "Fast_Ax_Amp_V"=w231) -> (w230:T17)
            n193 = Bundle By Name(cluster=w242, "Fast Axis Frequency (Hz)"=w253) -> (w252:T16)
            n194 = call "Volts to I16.vi"("Voltage (V)"=w231) -> ("I16"=w264:i16)  [unwired: 13 in, 1 out]
            n195 = call "Scan Parameters Action Engine.vi"("Action"=enum16{"Read", "Write"}."Write", "Scan Parameters IN"=w230) -> ()  [unwired: 13 in, 1 out]
            n196 = call "Manual Controls Action Engine.vi"("Action"=enum16{"Read", "Write"}."Read") -> ("Manual Controls Out"=w258:T18)  [unwired: 14 in]
            n197 = Bundle By Name(cluster=w258, "Res Mirror Amp (I16)"=w264, "Res Mirror Mute"=w250) -> (w256:T18)
            n198 = call "Image Aquisition Param Ctrl_AE.vi"("Action"=enum16{"READ", "WRITE"}."WRITE", "Image Acquisition Parameters In"=w252) -> ()  [unwired: 9 in, 1 out]
            n199 = call "FPGA-7842R-Control V2.vi"("Action"=FPGA-7842R-Reference."Set Res Mirror", "Manual Controls"=w256, "Initialize"=TRUE) -> ()  [unwired: 11 in, 2 out]
            n200 = call "Manual Controls Action Engine.vi"("Action"=enum16{"Read", "Write"}."Write", "Manual Controls In"=w256) -> ()  [unwired: 13 in, 1 out]
          }
          frame "Detectors" {
            n201 = call "Detectors Crl_AE.vi"("Action"=enum16{"READ", "WRITE"}."WRITE", "Detectors Parameters In"="Detectors") -> ()  [unwired: 9 in, 1 out]
          }
          frame "Laser Controls" {
            w341 = FALSE ("element")
            n202 = Unbundle By Name("Laser Controls") -> ("STED"=w347:bool, "650 nm"=w344:bool, "590 nm"=w345:bool, "485 nm"=w346:bool, "STED Power (V)"=w338:dbl, "Manual Control"=w330:bool)
            n203 = local read "Live"() -> (w333:bool)
            n204 = call "LASERs_ Crl_AE.vi"("Action"=enum16{"READ", "WRITE"}."WRITE", "Detectors Parameters In"="Laser Controls") -> ()  [unwired: 9 in, 1 out]
            n205 = Or(x=w333, y=w330) -> (x .or. y?=w332:bool)
            n206 = In Range and Coerce(upper limit=10.0, x=w338, lower limit=0.0) -> (coerced(x)=w335:dbl)  [unwired: 1 out]
            n207 = Build Array(w347, w344, w345, w346, w341, w341, w341, w341) -> (w343:bool[])
            n208 = case shown="True" w332 {
              tunnel: "Laser Controls" -> [_ w361]
              frame False {
              }
              frame True {
                n209 = call "FPGA-7842R-Control V2.vi"("Action"=FPGA-7842R-Reference."Laser Control", "Laser Controls"=w361, "Initialize"=TRUE) -> ()  [unwired: 11 in, 2 out]
              }
            }
            n210 = Boolean Array To Number(Boolean array=w343) -> (number=w342:u32)
            n211 = To Unsigned Byte Integer(number=w342) -> (unsigned 8bit integer=w340:u8)
            n212 = call "U8_To_U32.vi"("U8 IN"=w340) -> ("U32 OUT"=w339:u32)  [unwired: 13 in, 1 out]
            n213 = call "Volts to I16.vi"("Voltage (V)"=w335) -> ("I16"=w334:i16)  [unwired: 13 in, 1 out]
            n214 = case shown="False" w330 {
              tunnel: "Laser Controls" -> [w359 _]
              frame False {
                n215 = Unbundle By Name(w359) -> ("650 nm"=w356:bool, "590 nm"=w355:bool, "485 nm"=w354:bool)
                n216 = call "Detectors Crl_AE.vi"("Action"=enum16{"READ", "WRITE"}."READ") -> ("Detectors Parameters Out"=w357:T14)  [unwired: 10 in]
                n217 = Bundle By Name(cluster=w357, "Far Red (685/40 nm)"=w356, "Orange (624/40 nm)"=w355, "Green (525/50 nm)"=w354) -> (w353:T14)
                n218 = call "Detectors Crl_AE.vi"("Action"=enum16{"READ", "WRITE"}."WRITE", "Detectors Parameters In"=w353) -> ()  [unwired: 9 in, 1 out]
              }
              frame True {
              }
            }
            n219 = call "Scan Parameters Action Engine.vi"("Action"=enum16{"Read", "Write"}."Read") -> ("Scan Parameters OUT"=w350:T17)  [unwired: 14 in]
            n220 = Bundle By Name(cluster=w350, "Laser_States _U32"=w339, "775_AOM_Volt_I16"=w334) -> (w348:T17)
            n221 = call "Scan Parameters Action Engine.vi"("Action"=enum16{"Read", "Write"}."Write", "Scan Parameters IN"=w348) -> ()  [unwired: 13 in, 1 out]
          }
          frame "Shutters" {
            n222 = Unbundle By Name("Shutters") -> ("Upper Shutter"=w373:bool, "Lower Shutter"=w372:bool)
            n223 = Not(x=w373) -> (.not. x?=w364:bool)
            n224 = Not(x=w372) -> (.not. x?=w363:bool)
            n225 = call "Manual Controls Action Engine.vi"("Action"=enum16{"Read", "Write"}."Read") -> ("Manual Controls Out"=w368:T18)  [unwired: 14 in]
            n226 = Bundle By Name(cluster=w368, "Upper Shutter"=w364, "Lower Shutter"=w363) -> (w365:T18)
            n227 = call "Manual Controls Action Engine.vi"("Action"=enum16{"Read", "Write"}."Write", "Manual Controls In"=w365) -> ()  [unwired: 13 in, 1 out]
            n228 = call "FPGA-7842R-Control V2.vi"("Action"=FPGA-7842R-Reference."Shutter Control", "Manual Controls"=w365, "Initialize"=TRUE) -> ()  [unwired: 11 in, 2 out]
          }
        }
      }
      event Value Change {
        # "For P541 - Sample Z - Converting from Step in µm to I16 is as follows. We have (Step µw)*(10 V / 100 µm)*(32768 I16 / 10 V) = (Step µm)*(32768 I16 / 100 µm) = (Step µm)*(327.68 I16/µm)"
        n229 = event-data() -> ("CtlRef"=w387:refnum<vi>, "OldVal"=w385:variant, "NewVal"=w386:variant)  [unwired: 1 in]
        n230 = local write "Abort AllStage"(FALSE ("Abort AllStage")) -> ()
        n231 = property class="Clust"(reference=w387) -> ("Label.Text"=w384:string)  [unwired: 1 in, 2 out]
        n232 = case shown="\"Sample Z Coarse - M227\"" w384 {
          tunnel: w386 -> [_ w410 w451 w478 w541 w582 w611 w650]
          tunnel: w385 -> [_ w409 w450 w477 w542 w583 w612 w651]
          tunnel: ["" "N664" "ASI" "P612" "P612" "P841" "M227" "M686"] -> w383
          tunnel: [dbl[] [0.0] w401 w443 w466 dbl[] [0.0] w571 w604 w640] -> w382
          tunnel: [bool[] [FALSE] w399 w437 w467 bool[] [FALSE] bool[] [TRUE] w605 w639] -> w381
          tunnel: [enum16{"MOVE", "MVR"}."MVR" ("MOVE/MVR") w398 w440 w469 enum16{"MOVE", "MVR"}."MVR" ("MOVE/MVR") w574 w597 w642] -> w380
          tunnel: [0.0 ("Step Size (um)") 0.5 ("Step Size (um)") w442 0.0 ("Velocity") 0.0 ("Velocity") 10000.0 ("Velocity") 0.0 ("Velocity") 0.0 ("Velocity")] -> w376
          tunnel: [StageStates."MVR" ("Action") w396 w441 w470 StageStates."POSITION" ("Action") w575 w601 w643] -> w374
          frame Default {
          }
          frame "Upper Objective Z - N664" {
            n233 = call "N664_Ctrl_Index.vi"("OldVal"=w409, "NewVal"=w410) -> ("Control Ref OUT"=w408:refnum<vi>, "N664 Out"=w406:T5)  [unwired: 12 in]
            n234 = property class="Ctl"(reference=w408) -> ("Label.Text"=w407:string)  [unwired: 1 in, 2 out]
            n235 = Unbundle By Name(w406) -> ("Step Size (um)"=w405:dbl, "Position (mm)"=w404:dbl)
            n236 = case shown="\"Home\"" w407 {
              tunnel: w405 -> [_ w415 w418 _ _ _]
              tunnel: [0.0 ("Step Size (um)") w414 w418 w423 w425 w430] -> w402
              tunnel: w404 -> [_ _ _ w423 w425 _]
              tunnel: [enum16{"MOVE", "MVR"}."MVR" ("MOVE/MVR") enum16{"MOVE", "MVR"}."MVR" ("MOVE/MVR") enum16{"MOVE", "MVR"}."MVR" ("MOVE/MVR") enum16{"MOVE", "MVR"}."MOVE" ("MOVE/MVR") enum16{"MOVE", "MVR"}."MOVE" ("MOVE/MVR") enum16{"MOVE", "MVR"}."MOVE" ("MOVE/MVR")] -> w398
              tunnel: [StageStates."MVR" ("Action") StageStates."MVR" ("Action") StageStates."MVR" ("Action") StageStates."MOVE" ("Action") StageStates."MOVE" ("Action") StageStates."MOVE" ("Action")] -> w396
              frame Default {
              }
              frame "Up N664" {
                n237 = Negate(x=w415) -> (-x=w414:dbl)
              }
              frame "Down N664" {
              }
              frame "Position (mm)" {
              }
              frame "Save" {
                n238 = Build Array(w425) -> (w424:dbl[])
                n239 = call "Stage_position_ae.vi"("Position In"=w424, "StageID"="N664", "Enum"=enum16{"WRITE", "READ", "HOME", "SAVE HOME"}."SAVE HOME") -> ()  [unwired: 7 in, 2 out]
              }
              frame "Home" {
                n240 = call "Stage_position_ae.vi"("StageID"="N664", "Enum"=enum16{"WRITE", "READ", "HOME", "SAVE HOME"}."HOME") -> ("Position Out"=w432:dbl[])  [unwired: 8 in, 1 out]
                n241 = Index Array(array=w432, index=0) -> (element=w430:dbl)
              }
            }
            n242 = Build Array(w402) -> (w401:dbl[])
            n243 = Build Array(TRUE) -> (w399:bool[])
          }
          frame "Cavity Translation Z - ASI" {
            n244 = call "ASI_Ctrl_Index.vi"("NewVal"=w451, "OldVal"=w450) -> ("ASI out"=w447:T6, "Control Ref OUT"=w449:refnum<vi>)  [unwired: 8 in]
            n245 = property class="Ctl"(reference=w449) -> ("Label.Text"=w448:string)  [unwired: 1 in, 2 out]
            n246 = Unbundle By Name(w447) -> ("Step Size (um)"=w446:dbl, "Z (um)"=w445:dbl, "Velocity"=w442:dbl)
            n247 = case shown="\"Z (um)\"" w448 {
              tunnel: w446 -> [_ w457 w460 _]
              tunnel: w445 -> [_ _ _ w464]
              tunnel: [0.0 ("Z (um)") w457 w461 w464] -> w444
              tunnel: [StageStates."MVR" ("Action") StageStates."MVR" ("Action") StageStates."MVR" ("Action") StageStates."MOVE" ("Action")] -> w441
              tunnel: [enum16{"MOVE", "MVR"}."MVR" ("MOVE/MVR") enum16{"MOVE", "MVR"}."MVR" ("MOVE/MVR") enum16{"MOVE", "MVR"}."MVR" ("MOVE/MVR") enum16{"MOVE", "MVR"}."MOVE" ("MOVE/MVR")] -> w440
              frame Default {
              }
              frame "Up ASI" {
              }
              frame "Down ASI" {
                n248 = Negate(x=w460) -> (-x=w461:dbl)
              }
              frame "Z (um)" {
              }
            }
            n249 = Build Array(w444) -> (w443:dbl[])
            n250 = Build Array(TRUE) -> (w437:bool[])
          }
          frame "Bottom Objective XY - P612" {
            n251 = call "P612_Ctrl_Index.vi"("OldVal"=w477, "NewVal"=w478) -> ("Control out"=w476:refnum<vi>, "P612 out"=w474:T9)  [unwired: 12 in]
            n252 = property class="Ctl"(reference=w476) -> ("Label.Text"=w475:string)  [unwired: 1 in, 2 out]
            n253 = Unbundle By Name(w474) -> ("Step Size (um)"=w473:dbl, "X"=w472:dbl, "Y"=w471:dbl)
            n254 = case shown="\"Up Button\"" w475 {
              tunnel: w473 -> [_ _ w489 w496 w500 w507 _]
              tunnel: w472 -> [_ _ _ _ _ _ w514]
              tunnel: w471 -> [_ _ _ _ _ _ w513]
              tunnel: [StageStates."MVR" ("Action") StageStates."HOME" ("Action") StageStates."MVR" ("Action") StageStates."MVR" ("Action") StageStates."MVR" ("Action") StageStates."MVR" ("Action") StageStates."MOVE" ("Action")] -> w470
              tunnel: [enum16{"MOVE", "MVR"}."MVR" ("MOVE/MVR") enum16{"MOVE", "MVR"}."MVR" ("MOVE/MVR") enum16{"MOVE", "MVR"}."MVR" ("MOVE/MVR") enum16{"MOVE", "MVR"}."MVR" ("MOVE/MVR") enum16{"MOVE", "MVR"}."MVR" ("MOVE/MVR") enum16{"MOVE", "MVR"}."MVR" ("MOVE/MVR") enum16{"MOVE", "MVR"}."MOVE" ("MOVE/MVR")] -> w469
              tunnel: [bool[] [FALSE] bool[] [TRUE, TRUE] bool[] [TRUE, FALSE] bool[] [TRUE, FALSE] bool[] [FALSE, TRUE] bool[] [FALSE, TRUE] bool[] [TRUE, TRUE]] -> w467
              tunnel: [dbl[] [0.0] dbl[] [0.0, 0.0] w488 w495 w502 w509 w515] -> w466
              frame Default {
              }
              frame "Home Button" {
              }
              frame "Up Button" {
                n255 = Build Array(w489, 0.0 ("element")) -> (w488:dbl[])
              }
              frame "Down Button" {
                n256 = Negate(x=w496) -> (-x=w493:dbl)
                n257 = Build Array(w493, 0.0 ("element")) -> (w495:dbl[])
              }
              frame "Left Button" {
                n258 = Build Array(0.0 ("element"), w500) -> (w502:dbl[])
              }
              frame "Right Button" {
                n259 = Negate(x=w507) -> (-x=w506:dbl)
                n260 = Build Array(0.0 ("element"), w506) -> (w509:dbl[])
              }
              frame "X", "Y" {
                n261 = Build Array(w514, w513) -> (w515:dbl[])
              }
            }
          }
          frame "Sample Z - P541" {
            w520 = 327.68 ("y")
            n262 = call "P541_Ctrl_Index.vi"("OldVal"=w542, "NewVal"=w541) -> ("Control out"=w540:refnum<vi>, "P541 Out"=w539:T13)  [unwired: 12 in]
            n263 = Unbundle By Name(w539) -> ("Z Position"=w519:dbl, "Step Size (um)"=w538:dbl)
            n264 = property class="Ctl"(reference=w540) -> ("Label.Text"=w537:string)  [unwired: 1 in, 2 out]
            n265 = call "Manual Controls Action Engine.vi"("Action"=enum16{"Read", "Write"}."Read") -> ("Manual Controls Out"=w528:T18)  [unwired: 14 in]
            n266 = Unbundle By Name(w528) -> ("Z Axis Voltage (I16)"=w531:i16)
            n267 = Multiply(x=w519, y=w520) -> (x*y=w534:dbl)
            n268 = Multiply(x=w538, y=w520) -> (x*y=w536:dbl)
            n269 = Round To Nearest(number=w534) -> (nearest integer value=w523:dbl)
            n270 = Round To Nearest(number=w536) -> (nearest integer value=w522:dbl)
            n271 = To Word Integer(number=w523) -> (16bit integer=w533:i16)
            n272 = To Word Integer(number=w522) -> (16bit integer=w535:i16)
            n273 = case shown="\"Home\"" w537 {
              tunnel: w535 -> [_ w549 w553 _ _ _]
              tunnel: w533 -> [_ _ _ w555 _ _]
              tunnel: w531 -> [w548 w551 w554 _ w560 _]
              tunnel: [w548 w550 w552 w555 w560 w566] -> w527
              tunnel: w520 -> [_ _ _ _ _ w565]
              tunnel: w519 -> [_ _ _ _ w559 _]
              frame Default {
              }
              frame "Step Down" {
                n274 = Subtract(x=w551, y=w549) -> (x-y=w550:i16)
              }
              frame "Step Up" {
                n275 = Add(x=w554, y=w553) -> (x+y=w552:i16)
              }
              frame "Z Position" {
              }
              frame "Save" {
                n276 = Build Array(w559) -> (w558:dbl[])
                n277 = call "Stage_position_ae.vi"("Position In"=w558, "StageID"="P541", "Enum"=enum16{"WRITE", "READ", "HOME", "SAVE HOME"}."SAVE HOME") -> ()  [unwired: 7 in, 2 out]
              }
              frame "Home" {
                n278 = call "Stage_position_ae.vi"("StageID"="P541", "Enum"=enum16{"WRITE", "READ", "HOME", "SAVE HOME"}."HOME") -> ("Position Out"=w563:dbl[])  [unwired: 8 in, 1 out]
                n279 = Index Array(array=w563, index=0) -> (element=w561:dbl)
                n280 = Multiply(x=w561, y=w565) -> (x*y=w567:dbl)
                n281 = Round To Nearest(number=w567) -> (nearest integer value=w568:dbl)
                n282 = To Word Integer(number=w568) -> (16bit integer=w566:i16)
              }
            }
            n283 = Bundle By Name(cluster=w528, "Z Axis Voltage (I16)"=w527) -> (w530:T18)
            n284 = call "Manual Controls Action Engine.vi"("Action"=enum16{"Read", "Write"}."Write", "Manual Controls In"=w530) -> ("Manual Controls Out"=w524:T18)  [unwired: 13 in]
            n285 = call "FPGA-7842R-Control V2.vi"("Action"=FPGA-7842R-Reference."Stage Control", "Manual Controls"=w524, "Initialize"=TRUE) -> ()  [unwired: 11 in, 2 out]
          }
          frame "Phase Comp Mirror - P841" {
            n286 = call "P841_Ctrl_Index.vi"("OldVal"=w583, "NewVal"=w582) -> ("Control out"=w580:refnum<vi>, "P841 Out"=w578:T7)  [unwired: 12 in]
            n287 = property class="Ctl"(reference=w580) -> ("Label.Text"=w579:string)  [unwired: 1 in, 2 out]
            n288 = Unbundle By Name(w578) -> ("Position (µm)"=w577:dbl, "Step Size (µm)"=w576:dbl)
            n289 = case shown="Default" w579 {
              tunnel: w577 -> [_ _ _ w596]
              tunnel: w576 -> [_ w589 w593 _]
              tunnel: [0.0 ("Position (µm)") w589 w592 w596] -> w572
              tunnel: [StageStates."MVR" ("Action") StageStates."MVR" ("Action") StageStates."MVR" ("Action") StageStates."MOVE" ("Action")] -> w575
              tunnel: [enum16{"MOVE", "MVR"}."MVR" ("MOVE/MVR") enum16{"MOVE", "MVR"}."MVR" ("MOVE/MVR") enum16{"MOVE", "MVR"}."MVR" ("MOVE/MVR") enum16{"MOVE", "MVR"}."MOVE" ("MOVE/MVR")] -> w574
              frame Default {
              }
              frame "Up P841" {
              }
              frame "Down P841" {
                n290 = Negate(x=w593) -> (-x=w592:dbl)
              }
              frame "Position (µm)" {
              }
            }
            n291 = Build Array(w572) -> (w571:dbl[])
          }
          frame "Sample Z Coarse - M227" {
            n292 = call "M227_Ctrl_Index.vi"("OldVal"=w612, "NewVal"=w611) -> ("Control Ref OUT"=w610:refnum<vi>, "M227 Out"=w608:T11)  [unwired: 12 in]
            n293 = property class="Ctl"(reference=w610) -> ("Label.Text"=w609:string)  [unwired: 1 in, 2 out]
            n294 = Unbundle By Name(w608) -> ("Step Size (mm)"=w607:dbl, "MM 1"=w600:dbl, "MM 2"=w599:dbl, "MM 3"=w598:dbl)
            n295 = case shown="\"MM 1\"" w609 {
              tunnel: w607 -> [_ _ _ _ w631 w636]
              tunnel: [bool[] [FALSE, FALSE, FALSE] bool[] [TRUE, TRUE, TRUE] bool[] [TRUE, TRUE, TRUE] bool[] [TRUE, TRUE, TRUE] bool[] [TRUE, TRUE, TRUE] bool[] [TRUE, TRUE, TRUE]] -> w605
              tunnel: [0.0 ("Step Size (mm)") w618 w622 w626 w631 w635] -> w602
              tunnel: [StageStates."POSITION" ("Action") StageStates."MOVE" ("Action") StageStates."MOVE" ("Action") StageStates."MOVE" ("Action") StageStates."MVR" ("Action") StageStates."MVR" ("Action")] -> w601
              tunnel: w600 -> [_ w618 _ _ _ _]
              tunnel: w599 -> [_ _ w622 _ _ _]
              tunnel: w598 -> [_ _ _ w626 _ _]
              tunnel: [enum16{"MOVE", "MVR"}."MVR" ("MOVE/MVR") enum16{"MOVE", "MVR"}."MOVE" ("MOVE/MVR") enum16{"MOVE", "MVR"}."MOVE" ("MOVE/MVR") enum16{"MOVE", "MVR"}."MOVE" ("MOVE/MVR") enum16{"MOVE", "MVR"}."MVR" ("MOVE/MVR") enum16{"MOVE", "MVR"}."MVR" ("MOVE/MVR")] -> w597
              frame Default {
              }
              frame "MM 1" {
              }
              frame "MM 2" {
              }
              frame "MM 3" {
              }
              frame "Up M227" {
              }
              frame "Down M227" {
                n296 = Negate(x=w636) -> (-x=w635:dbl)
              }
            }
            n297 = Build Array(w602, w602, w602) -> (w604:dbl[])
          }
          frame "Sample Stage XY - M686" {
            n298 = call "M686_Ctrl_Index.vi"("NewVal"=w650, "OldVal"=w651) -> ("M686 - out"=w648:T8, "Control out"=w649:refnum<vi>)  [unwired: 8 in]
            n299 = Unbundle By Name(w648) -> ("Step Size (um)"=w647:dbl, "X"=w646:dbl, "Y"=w645:dbl)
            n300 = property class="Ctl"(reference=w649) -> ("Label.Text"=w638:string)  [unwired: 1 in, 2 out]
            n301 = case shown="\"Left Button\"" w638 {
              tunnel: w647 -> [_ _ w663 w668 w676 w681 _]
              tunnel: w646 -> [_ _ _ _ _ _ w688]
              tunnel: w645 -> [_ _ _ _ _ _ w687]
              tunnel: [StageStates."POSITION" ("Action") StageStates."MOVE" ("Action") StageStates."MVR" ("Action") StageStates."MVR" ("Action") StageStates."MVR" ("Action") StageStates."MVR" ("Action") StageStates."MOVE" ("Action")] -> w643
              tunnel: [enum16{"MOVE", "MVR"}."MVR" ("MOVE/MVR") enum16{"MOVE", "MVR"}."MOVE" ("MOVE/MVR") enum16{"MOVE", "MVR"}."MVR" ("MOVE/MVR") enum16{"MOVE", "MVR"}."MVR" ("MOVE/MVR") enum16{"MOVE", "MVR"}."MVR" ("MOVE/MVR") enum16{"MOVE", "MVR"}."MVR" ("MOVE/MVR") enum16{"MOVE", "MVR"}."MOVE" ("MOVE/MVR")] -> w642
              tunnel: [w653 dbl[] [12.5, 12.5] w661 w669 w677 w683 w689] -> w640
              tunnel: [bool[] [FALSE, FALSE] bool[] [TRUE, TRUE] bool[] [TRUE, TRUE] bool[] [TRUE, TRUE] bool[] [TRUE, TRUE] bool[] [TRUE, TRUE] bool[] [TRUE, TRUE]] -> w639
              frame Default {
                w654 = 0.0 ("Step Size (mm)")
                n302 = Build Array(w654, w654) -> (w653:dbl[])
              }
              frame "Home Button" {
              }
              frame "Right Button" {
                n303 = Build Array(w663, 0.0 ("element")) -> (w661:dbl[])
              }
              frame "Left Button" {
                n304 = Negate(x=w668) -> (-x=w667:dbl)
                n305 = Build Array(w667, 0.0 ("element")) -> (w669:dbl[])
              }
              frame "Up Button" {
                n306 = Negate(x=w676) -> (-x=w675:dbl)
                n307 = Build Array(0.0 ("element"), w675) -> (w677:dbl[])
              }
              frame "Down Button" {
                n308 = Build Array(0.0 ("element"), w681) -> (w683:dbl[])
              }
              frame "X", "Y" {
                n309 = Build Array(w688, w687) -> (w689:dbl[])
              }
            }
          }
        }
        n310 = case shown="Default" w384 {
          frame Default {
          }
          frame "Upper Objective Z - N664" {
            n311 = while {
              i -> [w698]
              stop <- w694 stop-if-true
              n312 = call "Stage_position_ae.vi"("StageID"="N664", "Enum"=enum16{"WRITE", "READ", "HOME", "SAVE HOME"}."READ") -> ("Status Out"=w695:bool, "Position Out"=w705:dbl[])  [unwired: 8 in]
              n313 = Greater?(x=w698, y=200) -> (0:w697:bool)
              n314 = And(x=w695, y=w697) -> (x .and. y?=w694:bool)
              n315 = Wait (ms)(milliseconds to wait=u32 1) -> ()  [unwired: 1 out]
              n316 = Index Array(array=w705, index=0) -> (element=w704:dbl)
              n317 = Select(t=u32 16777215, s=w694, f=u32 6618880) -> (s? t:f=w699:u32)
              n318 = property on="Position (mm)" class="DigNum (strict)"("Value"=w704, "NumText.BG Color"=w699) -> ()  [unwired: 2 in, 2 out]
            }
          }
          frame "Cavity Translation Z - ASI" {
            n319 = while {
              shift-right: [w712] -> _
              shift-left: TRUE ("Status Out") -> [w717]
              stop <- w716 stop-if-true
              n320 = call "Stage_position_ae.vi"("StageID"="ASI", "Enum"=enum16{"WRITE", "READ", "HOME", "SAVE HOME"}."READ") -> ("Status Out"=w712:bool, "Position Out"=w720:dbl[])  [unwired: 8 in]
              n321 = Greater?(x=w712, y=w717) -> (0:w716:bool)
              n322 = Wait (ms)(milliseconds to wait=u32 1) -> ()  [unwired: 1 out]
              n323 = Index Array(array=w720, index=0) -> (element=w710:dbl)
              n324 = Divide(x=w710, y=10.0) -> (x/y=w711:dbl)
              n325 = Select(t=u32 16777215, s=w712, f=u32 6618880) -> (s? t:f=w713:u32)
              n326 = property on="Z (um)" class="DigNum (strict)"("Value"=w711, "NumText.BG Color"=w713) -> ()  [unwired: 2 in, 2 out]
            }
          }
        }
        n327 = control-ref of="Abort AllStage"() -> (w375:refnum<vi>)
        n328 = call "AllStage_Limits_Array.vi"("Step(um)/Position(units)"=w382, "Axis"=w381, "Stage ID"=w383, "MOVE/MVR"=w380) -> ("Positions"=w378:dbl[], "Boolean Array"=w377:bool[], "Stage ID"=w379:string)  [unwired: 4 in, 1 out]
        n329 = call "AE_AllStages_Action V2.vi"("Velocity"=w376, "Abort"=w375, "Positions"=w378, "Axis"=w377, "Stage ID"=w379, "Action"=w374) -> ()  [unwired: 3 in, 3 out]
      }
      event "Stages": Value Change {
        n330 = event-data() -> ("NewVal"=w734:T10)  [unwired: 1 in, 2 out]
        n331 = Unbundle By Name(w734) -> ("M686"=w722:bool, "P841"=w732:bool, "ASI"=w730:bool, "N664"=w728:bool, "P612"=w726:bool, "M227"=w724:bool)
        n332 = call "All_Stages_Aloha.vi"("Aloha"=w722, "Stage ID"="M686") -> ()  [unwired: 9 in, 1 out]
        n333 = call "All_Stages_Aloha.vi"("Aloha"=w732, "Stage ID"="P841") -> ()  [unwired: 9 in, 1 out]
        n334 = call "All_Stages_Aloha.vi"("Aloha"=w730, "Stage ID"="ASI") -> ()  [unwired: 9 in, 1 out]
        n335 = call "All_Stages_Aloha.vi"("Aloha"=w728, "Stage ID"="N664") -> ()  [unwired: 9 in, 1 out]
        n336 = call "All_Stages_Aloha.vi"("Aloha"=w726, "Stage ID"="P612") -> ()  [unwired: 9 in, 1 out]
        n337 = call "All_Stages_Aloha.vi"("Aloha"=w724, "Stage ID"="M227") -> ()  [unwired: 9 in, 1 out]
      }
      event "SLM", "Timing", "DM", "Camera", "Focus Lock", "Stage Monitor": Value Change {
        n338 = event-data() -> ("CtlRef"=w738:refnum<vi>, "NewVal"=w735:bool)  [unwired: 1 in, 1 out]
        n339 = property class="Bool (strict)"(reference=w738) -> ("Label.Text"=w737:string)  [unwired: 1 in, 2 out]
        n340 = case shown="\"Focus Lock\"" w737 {
          tunnel: w735 -> [w739 w753 w767 w781 w794 w811]
          frame "SLM", Default {
            n341 = case shown="True" w739 {
              frame False {
                n342 = To Variant(anything=TRUE) -> (Variant=w745:variant)
                n343 = call "SLM AE.vi"("Action"=enum16{"READ", "WRITE"}."READ") -> ("SLM Ref Out"=w746:refnum<vi>)  [unwired: 10 in]
                n344 = invoke class="VI" method="Ctrl Val.Set"(reference=w746, "Control Name"="Exit", "Value"=w745) -> (reference out=w742:refnum<vi>, error out=w741:errorcluster)  [unwired: 2 in, 3 out]
                n345 = invoke on="Hamamatsu LCOS" class="SubPnl" method="Remove VI"(error in=w741) -> (error out=w740:errorcluster)  [unwired: 2 in, 2 out]
                n346 = Close Reference(reference=w742, error in (no error)=w740) -> ()  [unwired: 1 out]
              }
              frame True {
                n347 = Open VI Reference(vi path=path "C:/Users/ED STED/Documents/Test Control Software/Host VIs/SLM_V2/SLM Control.vi") -> (vi reference=w751:refnum<vi>)  [unwired: 5 in, 1 out]
                n348 = invoke class="VI" method="Run VI"(reference=w751, "Wait until done"=FALSE ("Wait Until Done")) -> (reference out=w748:refnum<vi>)  [unwired: 3 in, 4 out]
                n349 = invoke on="Hamamatsu LCOS" class="SubPanel" method="Insert VI"("VI Ref"=w748) -> ()  [unwired: 3 in, 4 out]
                n350 = call "SLM AE.vi"("Action"=enum16{"READ", "WRITE"}."WRITE", "SLM Ref In"=w748) -> ()  [unwired: 9 in, 1 out]
              }
            }
          }
          frame "DM" {
            n351 = case shown="False" w753 {
              frame False {
                n352 = call "DM_Ref_AE.vi"("Action"=enum16{"READ", "WRITE"}."READ") -> ("DM Ref Out"=w760:refnum<vi>)  [unwired: 10 in]
                n353 = To Variant(anything=TRUE) -> (Variant=w759:variant)
                n354 = invoke class="VI" method="Ctrl Val.Set"(reference=w760, "Control Name"="Exit", "Value"=w759) -> (reference out=w756:refnum<vi>, error out=w755:errorcluster)  [unwired: 2 in, 3 out]
                n355 = invoke on="BM Multi" class="SubPnl" method="Remove VI"(error in=w755) -> (error out=w754:errorcluster)  [unwired: 2 in, 2 out]
                n356 = Close Reference(reference=w756, error in (no error)=w754) -> ()  [unwired: 1 out]
              }
              frame True {
                n357 = Open VI Reference(vi path=path "C:/Users/ED STED/Documents/Test Control Software/Host VIs/DM_Dual_V2/Dual_DM_Control_Main_V4.vi") -> (vi reference=w765:refnum<vi>)  [unwired: 5 in, 1 out]
                n358 = invoke class="VI" method="Run VI"(reference=w765, "Wait until done"=FALSE ("Wait Until Done")) -> (reference out=w762:refnum<vi>)  [unwired: 3 in, 4 out]
                n359 = invoke on="BM Multi" class="SubPanel" method="Insert VI"("VI Ref"=w762) -> ()  [unwired: 3 in, 4 out]
                n360 = call "DM_Ref_AE.vi"("Action"=enum16{"READ", "WRITE"}."WRITE", "DM Ref In"=w762) -> ()  [unwired: 9 in, 1 out]
              }
            }
          }
          frame "Timing" {
            n361 = case shown="True" w767 {
              frame False {
                n362 = To Variant(anything=TRUE) -> (Variant=w772:variant)
                n363 = call "GateDelay AE.vi"("Action"=enum16{"READ", "WRITE"}."READ") -> ("Gate Delay Ref Out"=w773:refnum<vi>)  [unwired: 10 in]
                n364 = invoke class="VI" method="Ctrl Val.Set"(reference=w773, "Control Name"="Exit", "Value"=w772) -> (reference out=w768:refnum<vi>, error out=w769:errorcluster)  [unwired: 2 in, 3 out]
                n365 = invoke on="Timing" class="SubPnl" method="Remove VI"(error in=w769) -> (error out=w775:errorcluster)  [unwired: 2 in, 2 out]
                n366 = Close Reference(reference=w768, error in (no error)=w775) -> ()  [unwired: 1 out]
              }
              frame True {
                n367 = Open VI Reference(vi path=path "C:/Users/ED STED/Documents/Test Control Software/Host VIs/Time Delay/GateDelay_Control_V2.vi") -> (vi reference=w778:refnum<vi>)  [unwired: 5 in, 1 out]
                n368 = invoke class="VI" method="Run VI"(reference=w778, "Wait until done"=FALSE ("Wait Until Done")) -> (reference out=w777:refnum<vi>)  [unwired: 3 in, 4 out]
                n369 = invoke on="Timing" class="SubPanel" method="Insert VI"("VI Ref"=w777) -> ()  [unwired: 3 in, 4 out]
                n370 = call "GateDelay AE.vi"("Action"=enum16{"READ", "WRITE"}."WRITE", "Gate Delay Ref In"=w777) -> ()  [unwired: 9 in, 1 out]
              }
            }
          }
          frame "Camera" {
            n371 = case shown="False" w781 {
              frame False {
                n372 = To Variant(anything=TRUE) -> (Variant=w782:variant)
                n373 = call "Camera_Ref_HX.vi"("Action"=enum16{"READ", "WRITE"}."READ") -> ("Alignment Ref Out"=w786:refnum<vi>)  [unwired: 10 in]
                n374 = invoke class="VI" method="Ctrl Val.Set"(reference=w786, "Control Name"="Exit", "Value"=w782) -> (reference out=w785:refnum<vi>)  [unwired: 2 in, 4 out]
                n375 = invoke on="Tool Box" class="SubPnl" method="Remove VI"() -> (error out=w787:errorcluster)  [unwired: 3 in, 2 out]
                n376 = Close Reference(reference=w785, error in (no error)=w787) -> ()  [unwired: 1 out]
              }
              frame True {
                n377 = Open VI Reference(vi path=path "C:/Users/ED STED/Documents/Test Control Software/Host VIs/Camera/uEye_Control_V1.vi") -> (vi reference=w791:refnum<vi>)  [unwired: 5 in, 1 out]
                n378 = invoke class="VI" method="Run VI"(reference=w791, "Wait until done"=FALSE ("Wait Until Done")) -> (reference out=w790:refnum<vi>)  [unwired: 3 in, 4 out]
                n379 = invoke on="Tool Box" class="SubPnl" method="Insert VI"("VI Ref"=w790) -> ()  [unwired: 3 in, 4 out]
                n380 = call "Camera_Ref_HX.vi"("Action"=enum16{"READ", "WRITE"}."WRITE", "Alignment Ref In"=w790) -> ()  [unwired: 9 in, 1 out]
              }
            }
          }
          frame "Focus Lock" {
            n381 = case shown="True" w794 {
              frame False {
                n382 = call "Lock Control AE.vi"("Action"=Standard_Action_for_Focus_Lock."Read") -> ("Lock Control  out"=w797:T34)  [unwired: 1 in]
                n383 = Bundle By Name(cluster=w797, "EXIT"=TRUE) -> (w795:T34)
                n384 = call "FocusLock_Ref_HX.vi"("Action"=enum16{"READ", "WRITE"}."READ") -> ("FocusLock Ref Out"=w803:refnum<vi>)  [unwired: 10 in]
                n385 = To Variant(anything=w795) -> (Variant=w801:variant)
                n386 = invoke class="VI" method="Ctrl Val.Set"(reference=w803, "Control Name"="Lock Control", "Value"=w801) -> (reference out=w802:refnum<vi>, error out=w800:errorcluster)  [unwired: 2 in, 3 out]
                n387 = invoke on="Focus Lock\nFocus Lock Panel" class="SubPnl" method="Remove VI"(error in=w800) -> (error out=w804:errorcluster)  [unwired: 2 in, 2 out]
                n388 = Close Reference(reference=w802, error in (no error)=w804) -> ()  [unwired: 1 out]
              }
              frame True {
                n389 = Open VI Reference(vi path=path "C:/Users/ED STED/Documents/Test Control Software/Host VIs/Focus Lock/FocusLock Control v2.vi") -> (vi reference=w808:refnum<vi>)  [unwired: 5 in, 1 out]
                n390 = invoke class="VI" method="Run VI"(reference=w808, "Wait until done"=FALSE ("Wait Until Done")) -> (reference out=w807:refnum<vi>)  [unwired: 3 in, 4 out]
                n391 = invoke on="Focus Lock\nFocus Lock Panel" class="SubPnl" method="Insert VI"("VI Ref"=w807) -> ()  [unwired: 3 in, 4 out]
                n392 = call "FocusLock_Ref_HX.vi"("Action"=enum16{"READ", "WRITE"}."WRITE", "FocusLock Ref In"=w807) -> ()  [unwired: 9 in, 1 out]
              }
            }
          }
          frame "Stage Monitor" {
            n393 = case shown="True" w811 {
              frame False {
                n394 = call "StageMonitor_Ref_HX.vi"("Action"=enum16{"READ", "WRITE"}."READ") -> ("StageMonitor Ref Out"=w814:refnum<vi>)  [unwired: 10 in]
                n395 = To Variant(anything=TRUE) -> (Variant=w817:variant)
                n396 = invoke class="VI" method="Ctrl Val.Set"(reference=w814, "Control Name"="Exit", "Value"=w817) -> (reference out=w818:refnum<vi>, error out=w816:errorcluster)  [unwired: 2 in, 3 out]
                n397 = invoke on="Tool Box 2" class="SubPnl" method="Remove VI"(error in=w816) -> (error out=w819:errorcluster)  [unwired: 2 in, 2 out]
                n398 = Close Reference(reference=w818, error in (no error)=w819) -> ()  [unwired: 1 out]
              }
              frame True {
                n399 = Open VI Reference(vi path=path "C:/Users/ED STED/Documents/Test Control Software/Host VIs/Stages/Stage Monitor/Stage Monitor.vi") -> (vi reference=w822:refnum<vi>)  [unwired: 5 in, 1 out]
                n400 = invoke class="VI" method="Run VI"(reference=w822, "Wait until done"=FALSE ("Wait Until Done")) -> (reference out=w821:refnum<vi>)  [unwired: 3 in, 4 out]
                n401 = invoke on="Tool Box 2" class="SubPnl" method="Insert VI"("VI Ref"=w821) -> ()  [unwired: 3 in, 4 out]
                n402 = call "StageMonitor_Ref_HX.vi"("Action"=enum16{"READ", "WRITE"}."WRITE", "StageMonitor Ref In"=w821) -> ()  [unwired: 9 in, 1 out]
              }
            }
          }
        }
      }
      event Value Change {
        n403 = event-data() -> ("CtlRef"=w830:refnum<vi>, "OldVal"=w828:variant, "NewVal"=w827:variant)  [unwired: 1 in]
        n404 = property class="Clust"(reference=w830) -> ("Label.Text"=w829:string)  [unwired: 1 in, 2 out]
        n405 = call "Graph Ref AE.vi"("Action"=enum16{"READ", "WRITE"}."READ") -> ("Graph Ref Out"=w825:refnum<vi>[])  [unwired: 10 in]
        n406 = case shown="\"Graph Tools\"" w829 {
          tunnel: w828 -> [_ w837 w893]
          tunnel: w827 -> [_ w838 w892]
          tunnel: w825 -> [_ w832 w885]
          frame Default {
          }
          frame "Display Controls" {
            n407 = call "Display_Controls_Ctrl_Index.vi"("OldVal"=w837, "NewVal"=w838) -> ("Control Ref OUT"=w836:refnum<vi>, "Display Controls Out"=w834:T2)  [unwired: 12 in]
            n408 = property class="Ctl"(reference=w836) -> ("Label.Text"=w835:string)  [unwired: 1 in, 2 out]
            n409 = Unbundle By Name(w834) -> ("Single Screen"=w833:bool)
            n410 = case shown="\"Single Screen\", Default" w835 {
              tunnel: w833 -> [w846 _ _]
              tunnel: w832 -> [_ w871 w878]
              frame "Single Screen", Default {
                n411 = property class="App"() -> ("Disp.AllMonitors"=w845:T35)  [unwired: 2 in, 2 out]
                n412 = Index Array(array=w845, index #1=2 ("index"), index #2=0 ("index")) -> (element #1=w842:T36, element #2=w841:T36)
                n413 = control-ref of="This VI"() -> (w840:refnum<vi>)
                n414 = case shown="False" w846 {
                  tunnel: w842 -> [w850 _]
                  tunnel: w841 -> [w849 w861]
                  tunnel: w840 -> [w848 w859]
                  tunnel: T24 {"Left"=0, "Top"=0, "Right"=0, "Bottom"=0} ("Front Panel Window:Window Bounds") -> [w847 w860]
                  frame False {
                    w855 = i16 0
                    n415 = Unbundle By Name(w849) -> ("Bounds.Left"=w852:i16, "Bounds.Bottom"=w853:i16, "Bounds.Top"=w854:i16)
                    n416 = Unbundle By Name(w850) -> ("Bounds.Right"=w851:i16)
                    n417 = Subtract(x=w851, y=w852) -> (x-y=w856:i16)
                    n418 = Subtract(x=w853, y=w854) -> (x-y=w857:i16)
                    n419 = Bundle By Name(cluster=w847, "Left"=w855, "Top"=w855, "Right"=w856, "Bottom"=w857) -> (w858:T24)
                    n420 = property class="VI"(reference=w848, "Front Panel.WinBounds"=w858) -> ()  [unwired: 1 in, 2 out]
                  }
                  frame True {
                    w864 = i16 0
                    n421 = Unbundle By Name(w861) -> ("Bounds.Right"=w867:i16, "Bounds.Bottom"=w866:i16, "Bounds.Top"=w865:i16)
                    n422 = Subtract(x=w866, y=w865) -> (x-y=w863:i16)
                    n423 = Bundle By Name(cluster=w860, "Left"=w864, "Top"=w864, "Right"=w867, "Bottom"=w863) -> (w862:T24)
                    n424 = property class="VI"(reference=w859, "Front Panel.WinBounds"=w862) -> (reference out=w869:refnum<vi>)  [unwired: 1 in, 1 out]
                    n425 = property class="VI"(reference=w869, "FP.State"=T25."Maximized" ("Front Panel Window:State")) -> ()  [unwired: 1 in, 2 out]
                  }
                }
              }
              frame "Add Display" {
                w872 = u16 0 items=["Read", "Write"] ("Action")
                w876 = u16 1 items=["Read", "Write"] ("Action")
                n426 = property on="Add Display" class="Bool (strict)"("Value"=FALSE) -> ()  [unwired: 2 in, 2 out]
                n427 = call "Arange_Displays_V2.vi"("Action"=w872) -> ("Number of Channels OUT"=w873:i32)  [unwired: 14 in]
                n428 = Increment(x=w873) -> (x+1=w875:i32)
                n429 = call "Arange_Displays_V2.vi"("Display References"=w871, "Action"=w876, "Number of Channels"=w875, "Aspect Ratio (h/w)"=1.0) -> ()  [unwired: 11 in, 1 out]
              }
              frame "Remove Display" {
                w879 = u16 0 items=["Read", "Write"] ("Action")
                w883 = u16 1 items=["Read", "Write"] ("Action")
                n430 = call "Arange_Displays_V2.vi"("Action"=w879) -> ("Number of Channels OUT"=w880:i32)  [unwired: 14 in]
                n431 = Decrement(x=w880) -> (x-1=w882:i32)
                n432 = call "Arange_Displays_V2.vi"("Display References"=w878, "Action"=w883, "Number of Channels"=w882, "Aspect Ratio (h/w)"=1.0) -> ()  [unwired: 11 in, 1 out]
                n433 = property on="Remove Display" class="Bool (strict)"("Value"=FALSE) -> ()  [unwired: 2 in, 2 out]
              }
            }
          }
          frame "Graph Tools" {
            n434 = call "Graph_Controls_Ctrl_Index.vi"("OldVal"=w893, "NewVal"=w892) -> ("Control Ref OUT"=w891:refnum<vi>, "Graph Tools Out"=w890:T3)  [unwired: 12 in]
            n435 = property class="Ctl"(reference=w891) -> (reference out=w887:refnum<vi>, "Label.Text"=w886:string)  [unwired: 1 in, 1 out]
            n436 = Unbundle By Name(w890) -> ("Show Cursor"=w889:bool, "Auto Scale"=w888:bool, "Color Map"=w884:T37)
            n437 = case shown="\"Fit Tool\"" w886 {
              selector: w886 -> [_ _ _ w964 _ _ _ _]
              tunnel: w889 -> [_ w933 _ _ _ _ _ _]
              tunnel: w888 -> [_ _ w953 _ _ _ _ _]
              tunnel: w885 -> [w902 w932 w954 w957 w994 w1001 w1014 w1022]
              tunnel: w887 -> [_ _ _ _ _ _ _ _]
              tunnel: w886 -> [_ _ _ w959 _ _ _ _]
              tunnel: w884 -> [w905 _ _ _ _ _ _ _]
              frame "Apply Color" {
                n438 = control-ref of="This VI"() -> (w904:refnum<vi>)
                n439 = call "GetDisplayClick.vi"("Display REFs In"=w902, "Calling VI REF"=w904) -> ("Display Index"=w903:i32)  [unwired: 13 in]
                n440 = Index Array(array=w902, index=w903) -> (element=w901:refnum<vi>)
                n441 = property class="IntGraph (strict)"(reference=w901) -> (reference out=w897:refnum<vi>, error out=w894:errorcluster, "ZScale.Maximum"=w900:dbl)  [unwired: 1 in]
                n442 = case shown="\"Gray\"" w905 {
                  tunnel: [cluster{dbl, u32}[] [{0.0, 0}, {0.07843137254901933, 131072}, {0.15686274509805287, 196608}, {0.235294117647058, 327680}, {0.3137254901960773, 458752}, {0.39215686274509665, 589824}, {0.47058823529410176, 720896}, {0.5490196078431353, 851971}, {0.6274509803921546, 983043}, {0.705882352941174, 1114115}, {0.7843137254902075, 1245187}, {0.8627450980392268, 1376259}, {0.941176470588232, 1507331}, {1.0196078431372513, 1638403}, {1.0980392156862848, 1769475}, {1.1764705882353041, 1769479}, {1.2549019607843093, 2031623}, {1.3333333333333286, 2162695}, {1.4117647058823621, 2293767}, {1.4901960784313673, 2424839}, {1.5686274509803866, 2555911}, {1.647058823529406, 2686983}, {1.7254901960784395, 2818055}, {1.8039215686274588, 2949127}, {1.882352941176464, 3080203}, {1.9607843137254832, 3211275}, {2.0392156862745168, 3342347}, {2.117647058823522, 3473419}, {2.1960784313725554, 3604491}, {2.2745098039215605, 3735563}, {2.352941176470594, 3866635}, {2.431372549019599, 3867403}, {2.5098039215686327, 4129547}, {2.588235294117638, 4260619}, {2.6666666666666714, 4391691}, {2.7450980392156907, 4522763}, {2.823529411764696, 4653839}, {2.901960784313715, 4784911}, {2.9803921568627487, 4915983}, {3.058823529411768, 5178127}, {3.1372549019607874, 5309199}, {3.2156862745097925, 5440271}, {3.294117647058826, 5571343}, {3.3725490196078454, 5702415}, {3.4509803921568647, 5703439}, {3.52941176470587, 5965583}, {3.6078431372549034, 6096655}, {3.6862745098039227, 6227727}, {3.764705882352942, 6358799}, {3.8431372549019756, 6489871}, {3.9215686274509807, 6620943}, {4.0, 6752015}, {4.078431372549019, 6883087}, {4.1568627450980244, 7015183}, {4.235294117647058, 7146255}, {4.313725490196077, 7277327}, {4.392156862745097, 7408399}, {4.470588235294102, 7539471}, {4.549019607843135, 7670543}, {4.627450980392155, 7801615}, {4.705882352941174, 8063759}, {4.784313725490179, 8194831}, {4.862745098039213, 8326927}, {4.941176470588232, 8457999}, {5.019607843137251, 8589075}, {5.098039215686285, 8720147}, {5.17647058823529, 8851219}, {5.254901960784309, 8982291}, {5.333333333333329, 9113363}, {5.411764705882362, 9114387}, {5.490196078431367, 9376531}, {5.568627450980401, 9507603}, {5.647058823529406, 9638675}, {5.7254901960784395, 9769747}, {5.803921568627445, 9901843}, {5.882352941176478, 10032915}, {5.960784313725483, 10163987}, {6.039215686274517, 10229523}, {6.117647058823522, 10295059}, {6.196078431372555, 10427155}, {6.2745098039215605, 10558227}, {6.352941176470594, 10689299}, {6.431372549019599, 10820371}, {6.509803921568633, 10886931}, {6.588235294117638, 10952467}, {6.666666666666671, 11083539}, {6.745098039215691, 11214611}, {6.82352941176471, 11215635}, {6.901960784313715, 11477779}, {6.980392156862749, 11543315}, {7.058823529411768, 11608851}, {7.137254901960787, 11740947}, {7.215686274509821, 11806483}, {7.294117647058826, 11872019}, {7.372549019607845, 12004115}, {7.450980392156865, 12135187}, {7.529411764705898, 12266259}, {7.607843137254903, 12267283}, {7.686274509803923, 12398355}, {7.764705882352942, 12529427}, {7.843137254901947, 12530451}, {7.921568627450981, 12595987}, {8.0, 12530451}, {8.07843137254902, 12793619}, {8.156862745098024, 12794131}, {8.235294117647058, 12794643}, {8.313725490196077, 13056787}, {8.392156862745097, 13057299}, {8.47058823529413, 13057811}, {8.549019607843135, 13188883}, {8.627450980392155, 13320979}, {8.705882352941174, 13386515}, {8.784313725490179, 13452563}, {8.862745098039213, 13584147}, {8.941176470588232, 13584659}, {9.019607843137251, 13585171}, {9.098039215686256, 13585683}, {9.17647058823529, 13717267}, {9.254901960784323, 13848339}, {9.333333333333329, 13849363}, {9.411764705882362, 13849875}, {9.490196078431367, 13850387}, {9.5686274509804, 13981459}, {9.647058823529406, 14113555}, {9.72549019607844, 14114067}, {9.803921568627445, 14114579}, {9.882352941176478, 14115091}, {9.960784313725483, 14246675}, {10.039215686274517, 14377747}, {10.117647058823522, 14378771}, {10.196078431372555, 14379283}, {10.27450980392156, 14379539}, {10.352941176470594, 14379795}, {10.4313725490196, 14380819}, {10.509803921568633, 14511891}, {10.588235294117638, 14643987}, {10.666666666666671, 14644503}, {10.745098039215677, 14645015}, {10.82352941176471, 14645527}, {10.901960784313744, 14646039}, {10.980392156862749, 14646551}, {11.058823529411768, 14778135}, {11.137254901960787, 14909207}, {11.215686274509821, 14910231}, {11.294117647058826, 14910747}, {11.372549019607845, 14911259}, {11.450980392156865, 14911771}, {11.52941176470587, 14912283}, {11.607843137254903, 14912797}, {11.686274509803923, 15044383}, {11.764705882352942, 15175455}, {11.843137254901947, 15175967}, {11.92156862745098, 15176479}, {12.0, 15176991}, {12.07843137254902, 15177507}, {12.156862745098053, 15178019}, {12.235294117647058, 15178531}, {12.313725490196092, 15310115}, {12.392156862745097, 15441701}, {12.47058823529413, 15441959}, {12.549019607843135, 15442215}, {12.627450980392155, 15442727}, {12.705882352941174, 15443243}, {12.784313725490179, 15443755}, {12.862745098039213, 15444269}, {12.941176470588246, 15444783}, {13.019607843137251, 15444783}, {13.098039215686285, 15576367}, {13.17647058823529, 15707953}, {13.25490196078431, 15708467}, {13.333333333333329, 15708979}, {13.411764705882362, 15708981}, {13.490196078431367, 15708983}, {13.568627450980387, 15710011}, {13.647058823529406, 15710523}, {13.725490196078411, 15711037}, {13.803921568627459, 15711039}, {13.882352941176464, 15711553}, {13.960784313725512, 15843139}, {14.039215686274517, 15974213}, {14.117647058823522, 15974215}, {14.196078431372541, 15974217}, {14.27450980392156, 15974219}, {14.352941176470594, 15975755}, {14.431372549019613, 15976271}, {14.509803921568633, 15976785}, {14.588235294117666, 15977299}, {14.666666666666671, 15977301}, {14.745098039215677, 15977815}, {14.82352941176471, 15978327}, {14.901960784313744, 15978331}, {14.980392156862749, 16109917}, {15.058823529411768, 16241503}, {15.137254901960787, 16241505}, {15.215686274509792, 16242019}, {15.294117647058826, 16242535}, {15.372549019607845, 16242537}, {15.450980392156865, 16242539}, {15.529411764705898, 16243563}, {15.607843137254903, 16243567}, {15.686274509803908, 16244081}, {15.764705882352942, 16244595}, {15.843137254901947, 16244599}, {15.92156862745098, 16244601}, {16.0, 16244603}, {16.07843137254902, 16245627}, {16.156862745098024, 16245631}, {16.235294117647058, 16245633}, {16.313725490196077, 16246147}, {16.392156862745097, 16246663}, {16.47058823529413, 16377735}, {16.549019607843135, 16508811}, {16.62745098039217, 16508815}, {16.705882352941174, 16509839}, {16.78431372549018, 16509843}, {16.862745098039213, 16509845}, {16.941176470588232, 16509847}, {17.01960784313725, 16510361}, {17.098039215686256, 16510875}, {17.17647058823529, 16510879}, {17.25490196078431, 16510881}, {17.33333333333333, 16510883}, {17.411764705882362, 16511399}, {17.49019607843138, 16511911}, {17.568627450980387, 16511915}, {17.647058823529406, 16511917}, {17.72549019607844, 16511919}, {17.80392156862746, 16511923}, {17.882352941176464, 16512437}, {17.960784313725483, 16512951}, {18.03921568627449, 16512955}, {18.117647058823522, 16512957}, {18.19607843137254, 16512959}, {18.27450980392156, 16512961}, {18.352941176470594, 16512963}, {18.431372549019613, 16512967}, {18.509803921568633, 16513481}, {18.588235294117638, 16513995}, {18.66666666666667, 16513999}, {18.74509803921569, 16514001}, {18.82352941176471, 16514003}, {18.901960784313744, 16514005}, {18.98039215686275, 16514007}, {19.058823529411754, 16514011}, {19.137254901960787, 16514013}, {19.215686274509792, 16514015}, {19.294117647058826, 16514019}, {19.372549019607845, 16514021}, {19.450980392156865, 16514023}, {19.52941176470587, 16514027}, {19.607843137254918, 16514029}, {19.686274509803923, 16514031}, {19.764705882352942, 16514035}, {19.843137254901947, 16514037}, {19.921568627450995, 16514039}, {20.0, 16514043}] ("Z Scale.Marker Values[]") cluster{dbl, u32}[] [{0.0, 0}, {85.0, 16711680}, {108.0, 16729344}, {127.0, 16744192}, {132.0, 16747520}, {140.0, 16753920}, {157.0, 16766720}, {170.0, 16776960}, {245.0, 16777184}, {250.0, 16777200}, {255.0, 16777215}] ("Z Scale.Marker Values[]") cluster{dbl, u32}[] [{0.0, 0}, {255.0, 16777215}] ("Z Scale.Marker Values[]") cluster{dbl, u32}[] [{0.0, 0}, {255.0, 16711680}] ("Z Scale.Marker Values[]") cluster{dbl, u32}[] [{0.0, 0}, {255.0, 65280}] ("Z Scale.Marker Values[]") cluster{dbl, u32}[] [{0.0, 0}, {255.0, 255}] ("Z Scale.Marker Values[]") cluster{dbl, u32}[] [{0.0, 0}, {255.0, 65535}] ("Z Scale.Marker Values[]") cluster{dbl, u32}[] [{0.0, 0}, {255.0, 16711935}] ("Z Scale.Marker Values[]") cluster{dbl, u32}[] [{0.0, 0}, {255.0, 16776960}] ("Z Scale.Marker Values[]") cluster{dbl, u32}[] [{0.0, 0}, {170.0, 16711680}, {245.0, 16777184}, {250.0, 16777200}, {255.0, 16448250}] ("Z Scale.Marker Values[]") cluster{dbl, u32}[] [{0.0, 0}, {170.0, 65280}, {245.0, 16777184}, {250.0, 16777200}, {255.0, 16448250}] ("Z Scale.Marker Values[]") cluster{dbl, u32}[] [{0.0, 0}, {170.0, 255}, {245.0, 16777184}, {250.0, 16777200}, {255.0, 16448250}] ("Z Scale.Marker Values[]") cluster{dbl, u32}[] [{0.0, 0}, {1.0, 131072}, {2.0, 196608}, {3.0, 327680}, {4.0, 458752}, {5.0, 589824}, {6.0, 720896}, {7.0, 851971}, {8.0, 983043}, {9.0, 1114115}, {10.0, 1245187}, {11.0, 1376259}, {12.0, 1507331}, {13.0, 1638403}, {14.0, 1769475}, {15.0, 1769479}, {16.0, 2031623}, {17.0, 2162695}, {18.0, 2293767}, {19.0, 2424839}, {20.0, 2555911}, {21.0, 2686983}, {22.0, 2818055}, {23.0, 2949127}, {24.0, 3080203}, {25.0, 3211275}, {26.0, 3342347}, {27.0, 3473419}, {28.0, 3604491}, {29.0, 3735563}, {30.0, 3866635}, {31.0, 3867403}, {32.0, 4129547}, {33.0, 4260619}, {34.0, 4391691}, {35.0, 4522763}, {36.0, 4653839}, {37.0, 4784911}, {38.0, 4915983}, {39.0, 5178127}, {40.0, 5309199}, {41.0, 5440271}, {42.0, 5571343}, {43.0, 5702415}, {44.0, 5703439}, {45.0, 5965583}, {46.0, 6096655}, {47.0, 6227727}, {48.0, 6358799}, {49.0, 6489871}, {50.0, 6620943}, {51.0, 6752015}, {52.0, 6883087}, {53.0, 7015183}, {54.0, 7146255}, {55.0, 7277327}, {56.0, 7408399}, {57.0, 7539471}, {58.0, 7670543}, {59.0, 7801615}, {60.0, 8063759}, {61.0, 8194831}, {62.0, 8326927}, {63.0, 8457999}, {64.0, 8589075}, {65.0, 8720147}, {66.0, 8851219}, {67.0, 8982291}, {68.0, 9113363}, {69.0, 9114387}, {70.0, 9376531}, {71.0, 9507603}, {72.0, 9638675}, {73.0, 9769747}, {74.0, 9901843}, {75.0, 10032915}, {76.0, 10163987}, {77.0, 10229523}, {78.0, 10295059}, {79.0, 10427155}, {80.0, 10558227}, {81.0, 10689299}, {82.0, 10820371}, {83.0, 10886931}, {84.0, 10952467}, {85.0, 11083539}, {86.0, 11214611}, {87.0, 11215635}, {88.0, 11477779}, {89.0, 11543315}, {90.0, 11608851}, {91.0, 11740947}, {92.0, 11806483}, {93.0, 11872019}, {94.0, 12004115}, {95.0, 12135187}, {96.0, 12266259}, {97.0, 12267283}, {98.0, 12398355}, {99.0, 12529427}, {100.0, 12530451}, {101.0, 12595987}, {102.0, 12530451}, {103.0, 12793619}, {104.0, 12794131}, {105.0, 12794643}, {106.0, 13056787}, {107.0, 13057299}, {108.0, 13057811}, {109.0, 13188883}, {110.0, 13320979}, {111.0, 13386515}, {112.0, 13452563}, {113.0, 13584147}, {114.0, 13584659}, {115.0, 13585171}, {116.0, 13585683}, {117.0, 13717267}, {118.0, 13848339}, {119.0, 13849363}, {120.0, 13849875}, {121.0, 13850387}, {122.0, 13981459}, {123.0, 14113555}, {124.0, 14114067}, {125.0, 14114579}, {126.0, 14115091}, {127.0, 14246675}, {128.0, 14377747}, {129.0, 14378771}, {130.0, 14379283}, {131.0, 14379539}, {132.0, 14379795}, {133.0, 14380819}, {134.0, 14511891}, {135.0, 14643987}, {136.0, 14644503}, {137.0, 14645015}, {138.0, 14645527}, {139.0, 14646039}, {140.0, 14646551}, {141.0, 14778135}, {142.0, 14909207}, {143.0, 14910231}, {144.0, 14910747}, {145.0, 14911259}, {146.0, 14911771}, {147.0, 14912283}, {148.0, 14912797}, {149.0, 15044383}, {150.0, 15175455}, {151.0, 15175967}, {152.0, 15176479}, {153.0, 15176991}, {154.0, 15177507}, {155.0, 15178019}, {156.0, 15178531}, {157.0, 15310115}, {158.0, 15441701}, {159.0, 15441959}, {160.0, 15442215}, {161.0, 15442727}, {162.0, 15443243}, {163.0, 15443755}, {164.0, 15444269}, {165.0, 15444783}, {166.0, 15444783}, {167.0, 15576367}, {168.0, 15707953}, {169.0, 15708467}, {170.0, 15708979}, {171.0, 15708981}, {172.0, 15708983}, {173.0, 15710011}, {174.0, 15710523}, {175.0, 15711037}, {176.0, 15711039}, {177.0, 15711553}, {178.0, 15843139}, {179.0, 15974213}, {180.0, 15974215}, {181.0, 15974217}, {182.0, 15974219}, {183.0, 15975755}, {184.0, 15976271}, {185.0, 15976785}, {186.0, 15977299}, {187.0, 15977301}, {188.0, 15977815}, {189.0, 15978327}, {190.0, 15978331}, {191.0, 16109917}, {192.0, 16241503}, {193.0, 16241505}, {194.0, 16242019}, {195.0, 16242535}, {196.0, 16242537}, {197.0, 16242539}, {198.0, 16243563}, {199.0, 16243567}, {200.0, 16244081}, {201.0, 16244595}, {202.0, 16244599}, {203.0, 16244601}, {204.0, 16244603}, {205.0, 16245627}, {206.0, 16245631}, {207.0, 16245633}, {208.0, 16246147}, {209.0, 16246663}, {210.0, 16377735}, {211.0, 16508811}, {212.0, 16508815}, {213.0, 16509839}, {214.0, 16509843}, {215.0, 16509845}, {216.0, 16509847}, {217.0, 16510361}, {218.0, 16510875}, {219.0, 16510879}, {220.0, 16510881}, {221.0, 16510883}, {222.0, 16511399}, {223.0, 16511911}, {224.0, 16511915}, {225.0, 16511917}, {226.0, 16511919}, {227.0, 16511923}, {228.0, 16512437}, {229.0, 16512951}, {230.0, 16512955}, {231.0, 16512957}, {232.0, 16512959}, {233.0, 16512961}, {234.0, 16512963}, {235.0, 16512967}, {236.0, 16513481}, {237.0, 16513995}, {238.0, 16513999}, {239.0, 16514001}, {240.0, 16514003}, {241.0, 16514005}, {242.0, 16514007}, {243.0, 16514011}, {244.0, 16514013}, {245.0, 16514015}, {246.0, 16514019}, {247.0, 16514021}, {248.0, 16514023}, {249.0, 16514027}, {250.0, 16514029}, {251.0, 16514031}, {252.0, 16514035}, {253.0, 16514037}, {254.0, 16514039}, {255.0, 16514043}] ("Z Scale.Marker Values[]")] -> w896
                  tunnel: w900 -> [w907 w908 w910 w912 w914 w916 w918 w920 w922 w924 w926 w928 w931]
                  tunnel: [w907 w908 w910 w912 w914 w916 w918 w920 w922 w924 w926 w928 w931] -> w898
                  frame "System", Default {
                  }
                  frame "Fire" {
                    # "Fire"
                  }
                  frame "Gray" {
                    # "Grayscale"
                  }
                  frame "Red" {
                    # "Red"
                  }
                  frame "Green" {
                    # "Green"
                  }
                  frame "Blue" {
                    # "Blue"
                  }
                  frame "Cyan" {
                    # "Cyan"
                  }
                  frame "Magenta" {
                    # "Magenta"
                  }
                  frame "Yellow" {
                    # "Yellow"
                  }
                  frame "Red-White" {
                    # "Red-White"
                  }
                  frame "Green-White" {
                    # "Green-White"
                  }
                  frame "Blue-White" {
                    # "Blue-White"
                  }
                  frame "Glow" {
                  }
                }
                n443 = property on="Apply Color" class="Bool (strict)"(error in=w894, "Value"=FALSE) -> ()  [unwired: 1 in, 2 out]
                n444 = property class="IntGraph (strict)"(reference=w897, "ZScale.MarkerVals[]"=w896, "ZScale.High Color"=u32 255, "ZScale.Maximum"=w898) -> ()  [unwired: 1 in, 2 out]
              }
              frame "Show Cursor", Default {
                w936 = 2.0 ("y")
                n445 = Index Array(array=w932, index=0) -> (element=w944:refnum<vi>)
                n446 = property class="IntGraph (strict)"(reference=w944) -> ("Value"=w943:sgl[][])  [unwired: 1 in, 2 out]
                n447 = Array Size(array=w943) -> (size(s)=w942:i32[])
                n448 = To Double Precision Float(number=w942) -> (double precision float=w939:dbl[])
                n449 = Index Array(array=w939, index #1=0 ("index"), index #2=1 ("index")) -> (element #1=w938:dbl, element #2=w937:dbl)
                n450 = Divide(x=w938, y=w936) -> (x/y=w935:dbl)
                n451 = Divide(x=w937, y=w936) -> (x/y=w934:dbl)
                n452 = for {
                  tunnel: w932 -> [w946] mode=indexing
                  tunnel: w935 -> [w948]
                  tunnel: w934 -> [w947]
                  tunnel: w933 -> [w949]
                  n453 = property class="IntGraph (strict)"(reference=w946, "Cursor.Visible"=w949, "Cursor.Cursor X"=w948, "Cursor.Cursor Y"=w947) -> ()  [unwired: 1 in, 2 out]
                }
              }
              frame "Auto Scale" {
                n454 = Select(t=u8 2 ("Z Scale.Scale Fit"), s=w953, f=u8 0) -> (s? t:f=w950:u8)
                n455 = for {
                  tunnel: w954 -> [w956] mode=indexing
                  tunnel: w950 -> [w955]
                  n456 = property class="IntGraph (strict)"(reference=w956, "ZScale.ScaleFit"=w955) -> ()  [unwired: 1 in, 2 out]
                }
              }
              frame "Pan Tool", "Reset Zoom", "Zoom In", "Zoom Out" {
                n457 = case shown="\"Reset Zoom\"" w964 {
                  tunnel: [0 ("Palette:Active Tool") 6 ("Palette:Active Tool") 7 ("Palette:Active Tool") 1 ("Palette:Active Tool") 0 ("Palette:Active Tool")] -> w958
                  tunnel: w957 -> [_ _ _ _ w976]
                  frame Default {
                  }
                  frame "Zoom In" {
                  }
                  frame "Zoom Out" {
                  }
                  frame "Pan Tool" {
                  }
                  frame "Reset Zoom" {
                    n458 = property on="Reset Zoom" class="Bool (strict)"("Value"=FALSE) -> ()  [unwired: 2 in, 2 out]
                    n459 = for {
                      tunnel: w976 -> [w981] mode=indexing
                      tunnel: 5 ("Palette:Active Tool") -> [w980]
                      n460 = property class="IntGraph (strict)"(reference=w981, "ActPaletteTool"=w980) -> ()  [unwired: 1 in, 2 out]
                    }
                  }
                }
                n461 = control-ref of="Zoom In"() -> (w960:refnum<vi>)
                n462 = control-ref of="Zoom Out"() -> (w962:refnum<vi>)
                n463 = control-ref of="Pan Tool"() -> (w961:refnum<vi>)
                n464 = Build Array(w960, w962, w961) -> (w963:refnum<vi>[])
                n465 = for {
                  tunnel: w963 -> [w969] mode=indexing
                  tunnel: w959 -> [w967]
                  n466 = property class="Bool (strict)"(reference=w969) -> (reference out=w968:refnum<vi>, "Label.Text"=w966:string)  [unwired: 1 in, 1 out]
                  n467 = Equal?(x=w966, y=w967) -> (x = y?=w965:bool)
                  n468 = property class="Bool (strict)"(reference=w968, "Value"=w965) -> ()  [unwired: 1 in, 2 out]
                }
                n469 = for {
                  tunnel: w957 -> [w971] mode=indexing
                  tunnel: w958 -> [w970]
                  n470 = property class="IntGraph (strict)"(reference=w971, "ActPaletteTool"=w970) -> ()  [unwired: 1 in, 2 out]
                }
              }
              frame "Load File" {
                w991 = u16 1 items=["Get Image", "Load and Read File"] ("Action")
                n471 = control-ref of="This VI"() -> (w993:refnum<vi>)
                n472 = property on="Load File" class="Bool (strict)"("Value"=FALSE) -> ()  [unwired: 2 in, 2 out]
                n473 = call "GetDisplayClick.vi"("Display REFs In"=w994, "Calling VI REF"=w993) -> ("Display Index"=w982:i32)  [unwired: 13 in]
                n474 = call "OpenDBL.vi"("Action"=w991) -> ("Image"=w990:sgl[], "Dimensions (Z, Y, X, t)"=w989:i32[])  [unwired: 11 in, 2 out]
                n475 = Index Array(array=w989, index #1=1 ("index"), index #2=2 ("index")) -> (element #1=w986:i32, element #2=w985:i32)
                n476 = Reverse 1D Array(array=w990) -> (reversed array=w984:sgl[])
                n477 = Reshape Array(w984, w986, w985) -> (w983:sgl[][])
                n478 = Index Array(array=w994, index=w982) -> (element=w992:refnum<vi>)
                n479 = property class="IntGraph (strict)"(reference=w992, "Value"=w983) -> ()  [unwired: 1 in, 2 out]
              }
              frame "Fit Tool" {
                n480 = control-ref of="This VI"() -> (w1003:refnum<vi>)
                n481 = call "Image Aquisition Param Ctrl_AE.vi"("Action"=enum16{"READ", "WRITE"}."READ") -> ("Image Acquisition Parameters Out"=w998:T16)  [unwired: 10 in]
                n482 = call "GetDisplayClick.vi"("Display REFs In"=w1001, "Calling VI REF"=w1003) -> ("Display Index"=w1002:i32)  [unwired: 13 in]
                n483 = Index Array(array=w1001, index=w1002) -> (element=w1000:refnum<vi>)
                n484 = property class="IntGraph (strict)"(reference=w1000) -> ("Value"=w999:sgl[][])  [unwired: 1 in, 2 out]
                n485 = vi-ref "QuickProfile_V3.vi"() -> (w1006:refnum<vi>)
                n486 = property class="VI Interface Type 0"(reference=w1006) -> ("Path"=w1009:path)  [unwired: 1 in, 2 out]
                n487 = Unbundle By Name(w998) -> ("Pixel Size (nm)"=w1005:dbl[])
                n488 = Index Array(array=w1005, index=0) -> (element=w1012:dbl)
                n489 = Open VI Reference(type specifier VI Refnum (for type only)=w1006, vi path=w1009, options=128) -> (vi reference=w1007:refnum<vi>)  [unwired: 3 in, 1 out]
                n490 = call-by-ref "Start Asynchronous Call"(reference=w1007, "Image IN"=w999, "Pixel Size (nm)"=w1012) -> (reference out=w1010:refnum<vi>, error out=w997:errorcluster)  [unwired: 15 in]
                n491 = Close Reference(reference=w1010) -> ()  [unwired: 1 in, 1 out]
                n492 = property on="Fit Tool" class="Bool (strict)"(error in=w997, "Value"=FALSE) -> ()  [unwired: 1 in, 2 out]
              }
              frame "Smooth Tool" {
                n493 = vi-ref "SmoothTool.vi"() -> (w1017:refnum<vi>)
                n494 = property on="Smooth Tool" class="Bool (strict)"("Value"=FALSE) -> ()  [unwired: 2 in, 2 out]
                n495 = property class="VI Interface Type 1"(reference=w1017) -> ("Path"=w1019:path)  [unwired: 1 in, 2 out]
                n496 = control-ref of="This VI"() -> (w1015:refnum<vi>)
                n497 = Open VI Reference(type specifier VI Refnum (for type only)=w1017, vi path=w1019, options=128) -> (vi reference=w1018:refnum<vi>)  [unwired: 3 in, 1 out]
                n498 = call-by-ref "Start Asynchronous Call"(reference=w1018, "Calling VI REF"=w1015, "Display REFs In"=w1014) -> (reference out=w1016:refnum<vi>)  [unwired: 11 in, 1 out]
                n499 = Close Reference(reference=w1016) -> ()  [unwired: 1 in, 1 out]
              }
              frame "Merge Tool" {
                n500 = vi-ref "MergeTool - Cambridge.vi"() -> (w1025:refnum<vi>)
                n501 = property class="VI Interface Type 2"(reference=w1025) -> ("Path"=w1027:path)  [unwired: 1 in, 2 out]
                n502 = property on="Merge Tool" class="Bool (strict)"("Value"=FALSE) -> ()  [unwired: 2 in, 2 out]
                n503 = control-ref of="This VI"() -> (w1023:refnum<vi>)
                n504 = Open VI Reference(type specifier VI Refnum (for type only)=w1025, vi path=w1027, options=128) -> (vi reference=w1026:refnum<vi>)  [unwired: 3 in, 1 out]
                n505 = call-by-ref "Start Asynchronous Call"(reference=w1026, "VI Reference"=w1023, "Display References"=w1022) -> (reference out=w1024:refnum<vi>)  [unwired: 11 in, 1 out]
                n506 = Close Reference(reference=w1024) -> ()  [unwired: 1 in, 1 out]
              }
            }
          }
        }
      }
      event "Channel 1", "Channel 2", "Channel 3", "Channel 4", "Channel 5", "Channel 6": Mouse Down; "Channel 1", "Channel 2", "Channel 3", "Channel 4", "Channel 5", "Channel 6": Mouse Up {
        n507 = event-data() -> ("Type"=w1034:T26, "CtlRef"=w1031:refnum<vi>)  [unwired: 1 in, 5 out]
        n508 = Equal?(x=w1034, y=lveventtype."Mouse Down" ("Type")) -> (x = y?=w1032:bool)
        n509 = call "Graph Ref AE.vi"("Action"=enum16{"READ", "WRITE"}."READ") -> ("Graph Ref Out"=w1029:refnum<vi>[])  [unwired: 10 in]
        n510 = case shown="True" w1032 {
          tunnel: w1031 -> [w1037 w1055]
          tunnel: w1029 -> [w1036 w1054]
          frame False {
            n511 = property class="IntGraph (strict)"(reference=w1037) -> (reference out=w1041:refnum<vi>, "ActPaletteTool"=w1038:i32)  [unwired: 1 in, 1 out]
            n512 = Not Equal?(x=w1038, y=0) -> (x != y?=w1040:bool)
            n513 = case shown="False" w1040 {
              tunnel: w1041 -> [w1044 w1050]
              tunnel: w1036 -> [w1043 w1047]
              frame False {
                n514 = property class="IntGraph (strict)"(reference=w1044) -> ("Cursor.Cursor Position"=w1042:T38)  [unwired: 1 in, 2 out]
                n515 = for {
                  tunnel: w1043 -> [w1045] mode=indexing
                  tunnel: w1042 -> [w1046]
                  n516 = property class="IntGraph (strict)"(reference=w1045, "Cursor.Cursor Position"=w1046) -> ()  [unwired: 1 in, 2 out]
                }
              }
              frame True {
                n517 = property class="IntGraph (strict)"(reference=w1050) -> ("XScale.Range"=w1049:T39, "YScale.Range"=w1048:T39)  [unwired: 1 in, 2 out]
                n518 = for {
                  tunnel: w1049 -> [w1053]
                  tunnel: w1048 -> [w1052]
                  tunnel: w1047 -> [w1051] mode=indexing
                  n519 = property class="IntGraph (strict)"(reference=w1051, "XScale.Range"=w1053, "YScale.Range"=w1052) -> ()  [unwired: 1 in, 2 out]
                }
              }
            }
          }
          frame True {
            n520 = for {
              tunnel: w1054 -> [w1060] mode=indexing
              tunnel: w1055 -> [w1061]
              n521 = Equal?(x=w1060, y=w1061) -> (x = y?=w1059:bool)
              n522 = Select(t=T27 {"Left"=2431, "Top"=-324} ("Z Scale.Position"), s=w1059, f=T27 {"Left"=0, "Top"=0}) -> (s? t:f=w1056:T27)
              n523 = property class="IntGraph (strict)"(reference=w1060, "ZScale.Visible"=w1059, "ZScale.Position"=w1056) -> ()  [unwired: 1 in, 2 out]
            }
          }
        }
      }
      event "Exit": Value Change {
        n524 = event-data() -> ("CtlRef"=w1086:refnum<vi>, "NewVal"=w1088:bool)  [unwired: 1 in, 1 out]
        n525 = Release Notifier(notifier=w1081, force destroy? (F)=TRUE) -> ()  [unwired: 1 in, 3 out]
        n526 = property class="Bool"(reference=w1086) -> ("Label.Text"=w1085:string)  [unwired: 1 in, 2 out]
        n527 = call "SLM AE.vi"("Action"=enum16{"READ", "WRITE"}."READ") -> ("SLM Ref Out"=w1079:refnum<vi>)  [unwired: 10 in]
        n528 = call "DM_Ref_AE.vi"("Action"=enum16{"READ", "WRITE"}."READ") -> ("DM Ref Out"=w1077:refnum<vi>)  [unwired: 10 in]
        n529 = call "GateDelay AE.vi"("Action"=enum16{"READ", "WRITE"}."READ") -> ("Gate Delay Ref Out"=w1078:refnum<vi>)  [unwired: 10 in]
        n530 = Enqueue Element(queue=w1087, element=w1085) -> ()  [unwired: 2 in, 3 out]
        n531 = Build Array(w1079, w1077, w1078) -> (w1076:refnum<vi>[])
        n532 = call "Stage_position_ae.vi"("StageID"="N664", "Enum"=enum16{"WRITE", "READ", "HOME", "SAVE HOME"}."HOME") -> ("Position Out"=w1068:dbl[])  [unwired: 8 in, 1 out]
        n533 = call "Stage_position_ae.vi"("StageID"="P541", "Enum"=enum16{"WRITE", "READ", "HOME", "SAVE HOME"}."HOME") -> ("Position Out"=w1072:dbl[])  [unwired: 8 in, 1 out]
        n534 = for {
          tunnel: w1076 -> [w1093] mode=indexing
          n535 = Not A Number/Path/Refnum?(number/path/refnum=w1093) -> (NaN/Path/Refnum?=w1092:bool)
          n536 = case shown="False" w1092 {
            tunnel: w1093 -> [w1094 _]
            frame False {
              n537 = To Variant(anything=TRUE) -> (Variant=w1095:variant)
              n538 = invoke class="VI" method="Ctrl Val.Set"(reference=w1094, "Control Name"="Exit", "Value"=w1095) -> (reference out=w1098:refnum<vi>)  [unwired: 2 in, 4 out]
              n539 = Close Reference(reference=w1098) -> ()  [unwired: 1 in, 1 out]
            }
            frame True {
            }
          }
        }
        n540 = Index Array(array=w1068, index=0) -> (element=w1065:dbl)
        n541 = property on="Stages" class="Clust (strict)"() -> ("Controls[]"=w1075:refnum<vi>[])  [unwired: 2 in, 2 out]
        n542 = Index Array(array=w1072, index=0) -> (element=w1066:dbl)
        n543 = Build Array(w1066, w1065) -> (w1064:dbl[])
        n544 = for {
          tunnel: w1075 -> [w1091] mode=indexing
          n545 = property class="Ctl"(reference=w1091) -> ("Label.Text"=w1090:string)  [unwired: 1 in, 2 out]
          n546 = call "All_Stages_Aloha.vi"("Aloha"=FALSE, "Stage ID"=w1090) -> ()  [unwired: 9 in, 1 out]
        }
        n547 = call-poly <vilib>:"Write To Spreadsheet File.vi"("format (%.3f)"="%.4f", "1D data"=w1064, "file path (dialog if empty)"=path "C:/Users/ED STED/Documents/Test Control Software/Host VIs/Stages/Stage Positions/home position.csv") -> ()  [unwired: 5 in, 1 out]
      }
    }
  }
  n548 = call "Manual Controls Action Engine.vi"("Action"=enum16{"Read", "Write"}."Write", "Manual Controls In"=w27) -> ("Manual Controls Out"=w29:T18)  [unwired: 13 in]
  n549 = call "FPGA-7842R-Control V2.vi"("Action"=FPGA-7842R-Reference."Initialize", "Manual Controls"=w29, "Initialize"=FALSE) -> ("Initalized"=w11:bool)  [unwired: 11 in, 1 out]
  n550 = while {
    shift-right: [w1111] -> _
    shift-left: "Idle" -> [w1112]
    tunnel: w18 -> [w1108]
    shift-right: [w1106] -> _
    shift-left: w11 -> [w1107]
    tunnel: w1 -> [w1099]
    stop <- w1110 stop-if-true
    n551 = call "Image Aquisition Param Ctrl_AE.vi"("Action"=enum16{"READ", "WRITE"}."READ") -> ("Image Acquisition Parameters Out"=w1105:T16)  [unwired: 10 in]
    n552 = call "Detectors Crl_AE.vi"("Action"=enum16{"READ", "WRITE"}."READ") -> ("Detectors Parameters Out"=w1103:T14)  [unwired: 10 in]
    n553 = call "Manual Controls Action Engine.vi"("Action"=enum16{"Read", "Write"}."Read") -> ("Manual Controls Out"=w1100:T18)  [unwired: 14 in]
    n554 = case shown="\"Display\"" w1112 {
      selector: w1112 -> [_ _ _ w1145 _ _ _ _ _ _]
      tunnel: ["Exit" w1121 "Idle" ("name (unnamed)") "Arange Displays" ("name (unnamed)") "Start FPGA Acquisition" ("name (unnamed)") "Display" ("name (unnamed)") "Close Images" ("name (unnamed)") "Idle" "Stop Waveforms" ("name (unnamed)") "Start Waveforms" ("name (unnamed)")] -> w1111
      tunnel: [TRUE w1123 w1130 w1153 w1171 w1195 w1236 w1269 w1274 w1280] -> w1110
      tunnel: FALSE -> [_ w1123 w1130 w1153 w1171 w1195 w1236 w1269 w1274 w1280]
      tunnel: w1108 -> [_ w1122 _ _ _ _ _ _ _ _]
      tunnel: w1107 -> [w1117 w1120 w1131 w1151 w1168 w1193 w1234 w1267 w1275 w1281]
      tunnel: [w1116 w1120 w1131 w1151 w1168 w1189 w1234 w1266 w1275 w1281] -> w1106
      tunnel: w1105 -> [_ _ _ w1144 _ w1188 _ _ _ w1278]
      tunnel: w1103 -> [_ _ _ w1143 _ _ _ _ _ w1276]
      tunnel: w1100 -> [_ _ _ w1134 _ _ _ _ _ _]
      tunnel: w1099 -> [_ _ _ _ w1161 _ _ _ _ _]
      frame "Exit" {
        n555 = call "Graph Ref AE.vi"("Action"=enum16{"READ", "WRITE"}."READ") -> ("Graph Ref Out"=w1114:refnum<vi>[])  [unwired: 10 in]
        n556 = call "FPGA-7842R-Control V2.vi"("Action"=FPGA-7842R-Reference."Close FPGA", "Initialize"=w1117) -> ("Initalized"=w1116:bool)  [unwired: 12 in, 1 out]
        n557 = Close Reference(reference=w1114) -> ()  [unwired: 1 in, 1 out]
      }
      frame "Idle", Default {
        n558 = Dequeue Element(queue=w1122, timeout in ms (-1)=-1) -> (element=w1121:string)  [unwired: 1 in, 3 out]
      }
      frame "Close Images" {
        w1126 = u16 0 items=["Read", "Write"] ("Mode")
        w1127 = u16 0 items=["Write", "Read"] ("Mode")
        n559 = call "File Action V1.vi"("Mode"=w1126) -> ("Files Open"=w1125:bool)  [unwired: 12 in, 2 out]
        n560 = call "Image_Actions_V1.vi"("Mode"=w1127, "Action"="Trash Images") -> ()  [unwired: 12 in, 2 out]
        n561 = case shown="True" w1125 {
          frame False {
          }
          frame True {
            w1133 = u16 1 items=["Read", "Write"] ("Mode")
            n562 = call "File Action V1.vi"("Action"="Close Files", "Mode"=w1133) -> ()  [unwired: 11 in, 3 out]
          }
        }
      }
      frame "Capture", "Live" {
        w1149 = u16 0 items=["Write", "Read"] ("Mode")
        n563 = Cluster To Array(cluster=w1143) -> (array=w1141:bool[])
        n564 = Index Array(array=w1141, index=4) -> (element=w1138:bool)
        n565 = Boolean To (0,1)(Boolean=w1141) -> (0, 1=w1142:i16[])
        n566 = Add Array Elements(numeric array=w1142) -> (sum=w1139:i16)
        n567 = To Long Integer(number=w1139) -> (32bit integer=w1136:i32)
        n568 = Unbundle By Name(w1144) -> ("Image Format"=w1146:u16)
        n569 = Select(t=1, s=w1138, f=w1136) -> (s? t:f=w1135:i32)
        n570 = case shown="\"Capture\"" w1145 {
          tunnel: w1144 -> [_ w1156]
          tunnel: w1135 -> [_ w1155]
          tunnel: w1134 -> [_ w1154]
          frame Default {
          }
          frame "Capture" {
            w1159 = u16 1 items=["Read", "Write"] ("Mode")
            n571 = call "File Action V1.vi"("Action"="Open Files", "Mode"=w1159, "Image Acquisition Parameters"=w1156, "Manual Controls In"=w1154, "File Path IN"="Save File Path", "Number of Channels"=w1155) -> ("File Path OUT"=w1157:path)  [unwired: 7 in, 2 out]
            n572 = local write "Save File Path"(w1157) -> ()
          }
        }
        n573 = To Long Integer(number=w1146) -> (32bit integer=w1148:i32)
        n574 = Bundle(w1148, w1148) -> (w1147:cluster{i32, i32})  [unwired: 1 in]
        n575 = call "Image_Actions_V1.vi"("Image Size (Pixels)"=w1147, "Mode"=w1149, "Number of Channels"=w1135, "Action"="Create Images") -> ()  [unwired: 10 in, 2 out]
      }
      frame "Arange Displays" {
        w1166 = u16 1 items=["Write", "Read"] ("Mode")
        w1169 = u16 1 items=["Read", "Write"] ("Action")
        n576 = call "Image_Actions_V1.vi"("Mode"=w1166) -> ("Image REFs OUT"=w1167:T40[])  [unwired: 13 in, 1 out]
        n577 = call "Graph Ref AE.vi"("Action"=enum16{"READ", "WRITE"}."READ", "Graph Ref In"=w1161) -> ("Graph Ref Out"=w1163:refnum<vi>[])  [unwired: 9 in]
        n578 = Array Size(array=w1167) -> (size(s)=w1165:i32)
        n579 = call "Arange_Displays_V2.vi"("Display References"=w1163, "Action"=w1169, "Number of Channels"=w1165, "Aspect Ratio (h/w)"=1.0) -> ("Number of Channels OUT"=w1164:i32)  [unwired: 11 in]
        n580 = for {
          N: w1164 -> [_]
          tunnel: w1163 -> [w1173] mode=indexing
          tunnel: [w1176] -> _ mode=indexing
          i -> [w1174]
          n581 = property class="IntGraph (strict)"(reference=w1173) -> ("Label.Text"=w1178:string)  [unwired: 1 in, 2 out]
          n582 = Equal To 0?(x=w1174) -> (x = 0?=w1175:bool)
          n583 = case shown="True" w1175 {
            tunnel: w1173 -> [_ w1179]
            frame False {
            }
            frame True {
              n584 = property class="IntGraph (strict)"(reference=w1179, "ZScale.Visible"=TRUE ("Z Scale.Visible"), "ZScale.Position"=T27 {"Left"=2431, "Top"=-324} ("Z Scale.Position")) -> ()  [unwired: 1 in, 2 out]
            }
          }
          n585 = To Unsigned Word Integer(number=w1174) -> (unsigned 16bit integer=w1177:u16)
          n586 = Bundle("Label.Text"=w1178, w1177) -> (w1176:cluster{"Label.Text":string, u16})  [unwired: 1 in]
        }
        "Graph Ref Out" <- w1161
      }
      frame "Start Waveforms" {
        n587 = Unbundle By Name("Laser Controls 2") -> ("Laser On Time (Ticks)"=w1183:i8, "Laser Delay (Ticks)"=w1182:i8)
        n588 = call "Initialize Waveforms V4.vi"("Image Acquisition Parameters"=w1188) -> ("Waveform Data to FPGA"=w1194:T41)  [unwired: 14 in]
        n589 = Unbundle By Name(w1188) -> ("Scan Type"=w1187:enum16{"Sample Scanning", "Beam Scanning"})
        n590 = call "FPGA-7842R-Control V2.vi"("Waveform Data"=w1194, "Action"=FPGA-7842R-Reference."Start Waveforms", "Laser On Time (Ticks)"=w1183, "Image Acquisition Parameters"=w1188, "Initialize"=w1193, "Laser Delay (Ticks)"=w1182) -> ("Initalized"=w1190:bool)  [unwired: 8 in, 1 out]
        n591 = Equal?(x=w1187, y=enum16{"Sample Scanning", "Beam Scanning"}."Sample Scanning" ("Scan Type")) -> (x = y?=w1185:bool)
        n592 = case shown="True" w1185 {
          tunnel: w1190 -> [w1196 w1201]
          tunnel: [w1196 w1200] -> w1189
          frame False {
          }
          frame True {
            n593 = call "Scan Parameters Action Engine.vi"("Action"=enum16{"Read", "Write"}."Read") -> ("Scan Parameters OUT"=w1198:T17)  [unwired: 14 in]
            n594 = Unbundle By Name(w1198) -> ("Unused_Axis_I16"=w1197:i16)
            n595 = call "FPGA-7842R-Control V2.vi"("Action"=FPGA-7842R-Reference."Unused Axis I16", "Initialize"=w1201, "Unused Axis Offset (I16)"=w1197) -> ("Initalized"=w1200:bool)  [unwired: 11 in, 1 out]
          }
        }
      }
      frame "Display" {
        w1229 = u16 1 items=["Write", "Read"] ("Mode")
        n596 = call "Image_Actions_V1.vi"("Mode"=w1229) -> ("Image REFs OUT"=w1231:T40[])  [unwired: 13 in, 1 out]
        n597 = Array Size(array=w1231) -> (size(s)=w1227:i32)
        n598 = Decrement(x=w1227) -> (x-1=w1226:i32)
        n599 = for {
          N: 6 -> [_]
          tunnel: w1226 -> [w1264]
          tunnel: [w1262] -> w1230 mode=indexing
          i -> [w1263]
          n600 = Greater Or Equal?(x=w1264, y=w1263) -> (x >= y?=w1262:bool)
        }
        n601 = Obtain Notifier(name (unnamed)="Running", notification data type=FALSE) -> (notifier out=w1203:refnum<notifier>)  [unwired: 2 in, 2 out]
        n602 = Index Array(array=w1230, index #1=1 ("index"), index #2=2 ("index"), index #3=3 ("index"), index #4=4 ("index"), index #5=5 ("index")) -> (element #1=w1215:bool, element #2=w1214:bool, element #3=w1213:bool, element #4=w1212:bool, element #5=w1211:bool)
        n603 = Index Array(array=w1231, index #1=0 ("index"), index #2=1 ("index"), index #3=2 ("index"), index #4=3 ("index"), index #5=4 ("index"), index #6=5 ("index")) -> (element #1=w1210:T40, element #2=w1209:T40, element #3=w1208:T40, element #4=w1207:T40, element #5=w1206:T40, element #6=w1205:T40)
        n604 = while {
          tunnel: w1215 -> [w1251]
          tunnel: w1214 -> [w1250]
          tunnel: w1213 -> [w1246]
          tunnel: w1212 -> [w1243]
          tunnel: w1211 -> [w1242]
          tunnel: w1210 -> [w1249]
          tunnel: w1209 -> [w1248]
          tunnel: w1208 -> [w1247]
          tunnel: w1207 -> [w1245]
          tunnel: w1206 -> [w1241]
          tunnel: w1205 -> [w1244]
          tunnel: w1203 -> [w1238]
          stop <- w1239 stop-if-true
          n605 = Get Notifier Status(notifier=w1238) -> (current notification=w1239:bool)  [unwired: 1 in, 4 out]
          n606 = case shown="False" w1251 {
            tunnel: w1248 -> [_ w1261]
            frame False {
            }
            frame True {
              n607 = call "IMAQ ImageToArray"("Image"=w1261) -> ("Image Pixels (Float)"=→"Channel 2":sgl[][])  [unwired: 3 in, 4 out]
            }
          }
          n608 = case shown="False" w1250 {
            tunnel: w1247 -> [_ w1259]
            frame False {
            }
            frame True {
              n609 = call "IMAQ ImageToArray"("Image"=w1259) -> ("Image Pixels (Float)"=→"Channel 3":sgl[][])  [unwired: 3 in, 4 out]
            }
          }
          n610 = call "IMAQ ImageToArray"("Image"=w1249) -> ("Image Pixels (Float)"=→"Channel 1":sgl[][])  [unwired: 3 in, 4 out]
          n611 = case shown="False" w1246 {
            tunnel: w1245 -> [_ w1257]
            frame False {
            }
            frame True {
              n612 = call "IMAQ ImageToArray"("Image"=w1257) -> ("Image Pixels (Float)"=→"Channel 4":sgl[][])  [unwired: 3 in, 4 out]
            }
          }
          n613 = case shown="False" w1243 {
            tunnel: w1241 -> [_ w1255]
            frame False {
            }
            frame True {
              n614 = call "IMAQ ImageToArray"("Image"=w1255) -> ("Image Pixels (Float)"=→"Channel 5":sgl[][])  [unwired: 3 in, 4 out]
            }
          }
          n615 = case shown="False" w1242 {
            tunnel: w1244 -> [_ w1253]
            frame False {
            }
            frame True {
              n616 = call "IMAQ ImageToArray"("Image"=w1253) -> ("Image Pixels (Float)"=→"Channel 6":sgl[][])  [unwired: 3 in, 4 out]
            }
          }
          n617 = Wait (ms)(milliseconds to wait=u32 100) -> ()  [unwired: 1 out]
        }
      }
      frame "Stop Waveforms" {
        n618 = call "FPGA-7842R-Control V2.vi"("Action"=FPGA-7842R-Reference."Stop Waveforms", "Initialize"=w1267) -> ("Initalized"=w1266:bool)  [unwired: 12 in, 1 out]
      }
      frame "Stop Acquisition" {
        n619 = call "FPGA-7842R-Control V2.vi"("Action"=FPGA-7842R-Reference."Laser Control", "Laser Controls"=T15 {"STED Power (V)"=0.0, "STED"=FALSE, "650 nm"=FALSE, "590 nm"=FALSE, "485 nm"=FALSE, "Manual Control"=FALSE} ("Laser Controls 2"), "Initialize"=TRUE) -> ()  [unwired: 11 in, 2 out]
      }
      frame "Start FPGA Acquisition" {
        n620 = Unbundle By Name(w1278) -> ("Scan Mode"=w1277:enum16{"XY", "XZ", "YZ", "XYZ"})
        n621 = case shown="\"XZ\", Default" w1277 {
          tunnel: w1278 -> [_ w1289]
          tunnel: w1276 -> [_ w1288]
          frame "YZ" {
            n622 = vi-ref "FPGA Sample Scanning V1.vi"() -> (w1284:refnum<vi>)
            n623 = property class="VI Interface Type 3"(reference=w1284) -> ("Path"=w1282:path)  [unwired: 1 in, 2 out]
            n624 = Open VI Reference(type specifier VI Refnum (for type only)=w1284, vi path=w1282, options=128) -> (vi reference=w1285:refnum<vi>)  [unwired: 3 in, 1 out]
            n625 = call-by-ref "Start Asynchronous Call"(reference=w1285) -> (reference out=w1286:refnum<vi>)  [unwired: 4 in, 1 out]
            n626 = Close Reference(reference=w1286) -> ()  [unwired: 1 in, 1 out]
          }
          frame "XZ", Default {
            n627 = vi-ref "FPGA Beam Scanning V2.vi"() -> (w1291:refnum<vi>)
            n628 = property class="VI Interface Type 4"(reference=w1291) -> ("Path"=w1292:path)  [unwired: 1 in, 2 out]
            n629 = Open VI Reference(type specifier VI Refnum (for type only)=w1291, vi path=w1292, options=128) -> (vi reference=w1290:refnum<vi>)  [unwired: 3 in, 1 out]
            n630 = call-by-ref "Start Asynchronous Call"(reference=w1290, "Detectors"=w1288, "Image Acquisition Parameters"=w1289) -> (reference out=w1287:refnum<vi>)  [unwired: 3 in, 1 out]
            n631 = Close Reference(reference=w1287) -> ()  [unwired: 1 in, 1 out]
          }
        }
      }
    }
  }
